vi "RTS Client.vi"() -> ()   [LabVIEW 2016]
uses:
  Type Definitions/RTS TDMS Filename Locations.ctl
  Type Definitions/RTS Save References.ctl
  Type Definitions/RTS Configuration Setup.ctl
  Type Definitions/RTS Wago Config.ctl
  Type Definitions/RTS APLUS Config.ctl
  Type Definitions/RTS Yokogawa MX Config.ctl
  Type Definitions/RTS Replay Server Control.ctl
  Type Definitions/RTS Server Configuration.ctl
  Type Definitions/RTS Station Settions TCP Comms.ctl
  Type Definitions/RTS Chamber Save Status.ctl
  Type Definitions/RTS Test Pattern.ctl
  Drivers/WAGO 750-881/Type Definitions/Wago Door Settings.ctl
  Drivers/WAGO 750-881/Type Definitions/Wago Door Relays By Station.ctl
  Drivers/WAGO 750-881/Type Definitions/Wago Door Operation.ctl
  Type Definitions/RTS Enable Door Openers.ctl
  Drivers/WAGO 750-881/Type Definitions/Wago Ground Leakage Relays.ctl
  Drivers/WAGO 750-881/Type Definitions/Wago Ground Leakage.ctl
  Drivers/WAGO 750-881/Type Definitions/Wago Polarity Selector Relays.ctl
  Drivers/WAGO 750-881/Type Definitions/Wago Polarity Selector.ctl
  Type Definitions/RTS Frequency Selector.ctl
  Drivers/WAGO 750-881/Type Definitions/Wago Room Enable.ctl
  Drivers/WAGO 750-881/Type Definitions/Wago Room Run.ctl
  Type Definitions/RTS Chamber Temperature Humidity Control.ctl
  Utility/Save File/File Setup (Public)/Type Definition/Save File DOE File Path Control.ctl
  Utility/Save File/File Setup (Public)/Type Definition/Save File DOE Data Save Filepaths.ctl
  Type Definitions/RTS Room Selector.ctl
  Type Definitions/RTS Reset Watt Hours.ctl
  Drivers/WAGO 750-881/Type Definitions/Wago Door Relays.ctl
  Drivers/WAGO 750-881/Type Definitions/Wago Contactor Settings.ctl
  Type Definitions/RTS TCP Commands.ctl
  Type Definitions/RTS TCP Multiple Connections Data.ctl
  Utility/Save File/File Setup (Public)/Type Definition/Save File DOE Configuration State.ctl
  Utility/Save File/File Setup (Public)/Type Definition/Save File DOE LabView Program.ctl
  Type Definitions/RTS Select System Number.ctl
  Utility/Save File/File Setup.lvlib
panel:
  in  "Custom CMD State":string
  in  "Test Setup":bool
  in  "Room Status":i32[](listbox)
  in  "Tree Selection":T1="Select Room/Stall"
  in  "Tab Control 3":enum32{"Page 1", "Page 2", "Page 3"}(tab)
  out "Start UI Loop":bool
  out "Raw Command":string
  in  "Filepath":T2
  out "Base Path":path
  out "Setup Info":string
  out "Data File Path":path
  out "Latest Save State":bool
  in  "Room OK?":T4
  in  "Room Run":T5
  out "Chamber Data":string[][](array[string])
  out "System Exit":bool=TRUE
  out "Control Exit":bool=TRUE
  out "Debug array 2":string[](array[string])
  in  "Debug?":bool
  out "Debug array":string[](array[string])
  out "Test Selected?":bool
  out "Point File Selected?":bool
  out "File Name Selected?":bool
  out "Deselect Log Data":bool=TRUE
  out "RTS Config Setup Output":T6
  in  "Tab Control 2":T15(tab)
  out "Chamber 1 Socket":string[][](array[string])
  out "Chamber 2 Socket":string[][](array[string])
  out "Chamber 3 Socket":string[][](array[string])
  out "Chamber 4 Socket":string[][](array[string])
  out "File  Version":string="Parametric Stand"
  in  "Save Data":bool
  out "Point File Path":path
  out "Error Out":errorcluster
  in  "Error In":errorcluster
  in  "Multicolumn Listbox":i32[](listbox)
  in  "Server Closed":string="The server VI closed the connection."
  in  "Configure Point File":bool
  in  "Setup Test":bool
  in  "Tab Control":T16(tab)
  out "Mixed Signal Graph 2":T17(graph)
  out "Tree Selection Display":string
  out "Save Status":T13
  in  "Wh Reset 8":T18 caption="Wh Reset"
  in  "Frequency 8":T19 caption="Frequency" items=["60 Hz", "50 Hz"]
  in  "Voltage 8":dbl caption="Voltage"
  in  "Wh Reset 7":T18 caption="Wh Reset"
  in  "Frequency 7":T19 caption="Frequency" items=["60 Hz", "50 Hz"]
  in  "Voltage 7":dbl caption="Voltage"
  in  "Wh Reset 6":T18 caption="Wh Reset"
  in  "Frequency 6":T19 caption="Frequency" items=["60 Hz", "50 Hz"]
  in  "Voltage 6":dbl caption="Voltage"
  in  "Wh Reset 5":T18 caption="Wh Reset"
  in  "Frequency 5":T19 caption="Frequency" items=["60 Hz", "50 Hz"]
  in  "Voltage 5":dbl caption="Voltage"
  in  "Wh Reset 4":T18 caption="Wh Reset"
  in  "Frequency 4":T19 caption="Frequency" items=["60 Hz", "50 Hz"]
  in  "Voltage 4":dbl caption="Voltage"
  in  "Wh Reset 3":T18 caption="Wh Reset"
  in  "Frequency 3":T19 caption="Frequency" items=["60 Hz", "50 Hz"]
  in  "Voltage 3":dbl caption="Voltage"
  in  "Wh Reset 2":T18 caption="Wh Reset"
  in  "Frequency 2":T19 caption="Frequency" items=["60 Hz", "50 Hz"]
  in  "Voltage 2":dbl caption="Voltage"
  in  "Wh Reset 1":T18 caption="Wh Reset"
  in  "Frequency":T19 items=["60 Hz", "50 Hz"]
  in  "Voltage":dbl
  in  "Station Voltage Send 5":bool
  in  "Station Voltage Send 1":bool
  in  "Station Voltage Send 6":bool
  in  "Station Voltage Send 2":bool
  in  "Station Voltage Send 7":bool
  in  "Station Voltage Send 3":bool
  in  "Station Voltage Send 8":bool
  in  "Station Voltage Send 4":bool
  in  "Polarity Selector":T20
  in  "Ground Leak Relays":T22
  out "Current Contactor Settings":T24
  out "Current Door Output Relays Status":T25
  in  "Station 8 CMD":bool
  in  "Station 7 CMD":bool
  in  "Station 6 CMD":bool
  in  "Station 5 CMD":bool
  in  "Station 4 CMD":bool
  in  "Station 3 CMD":bool
  in  "Station 2 CMD":bool
  in  "Station 1 CMD":bool
  in  "Door Settings":T26={"Station 1"={"Freezer"=enum."Clear Time Close Door", "Cab"=enum."Clear Time Close Door", "Slide"=enum."Clear Time Close Door"}, "Station 2"={"Freezer"=enum."Clear Time Close Door", "Cab"=enum."Clear Time Close Door", "Slide"=enum."Clear Time Close Door"}, "Station 3"={"Freezer"=enum."Clear Time Close Door", "Cab"=enum."Clear Time Close Door", "Slide"=enum."Clear Time Close Door"}, "Station 4"={"Freezer"=enum."Clear Time Close Door", "Cab"=enum."Clear Time Close Door", "Slide"=enum."Clear Time Close Door"}, "Station 5"={"Freezer"=enum."Clear Time Close Door", "Cab"=enum."Clear Time Close Door", "Slide"=enum."Clear Time Close Door"}, "Station 6"={"Freezer"=enum."Clear Time Close Door", "Cab"=enum."Clear Time Close Door", "Slide"=enum."Clear Time Close Door"}, "Station 7"={"Freezer"=enum."Clear Time Close Door", "Cab"=enum."Clear Time Close Door", "Slide"=enum."Clear Time Close Door"}, "Station 8"={"Freezer"=enum."Clear Time Close Door", "Cab"=enum."Clear Time Close Door", "Slide"=enum."Clear Time Close Door"}, "Door Enable"=enum."Enable Door Openers"}
  in  "Room Setpoints":T30={"Room Setpoint Temperature (*RM Dry Set P1)"=90.0, "Room Setpoint Humidity (*RM Hum Set P1)"=20.0, "Room Cool Temperature (*RM Cool Setp 1)"=65.0, "Room Dehum Temperature (*RM De Hum Set P1)"=60.0} {"Room Dehum Temperature (*RM De Hum Set P1)" min=30.0 max=120.0; "Room Cool Temperature (*RM Cool Setp 1)" min=30.0 max=120.0; "Room Setpoint Humidity (*RM Hum Set P1)" min=5.0 max=98.0; "Room Setpoint Temperature (*RM Dry Set P1)" min=40.0 max=120.0}
  in  "Update Room Setpoint":bool
  in  "CSV Data Save":T31={"CSV File Location"=path "C:/Technology Lab/NI-2010/Trunk/Refrigeration/RTS/System_Test_Data1.tdms", "CSV File Location 2"=path "C:/Technology Lab/NI-2010/Trunk/Refrigeration/RTS/System_Test_Data1.tdms", "CSV File Location 3"=path "", "CSV File Location 4"=path "", "CSV File Location 5"=path "", "CSV File Location 6"=path "", "CSV File Location 7"=path "", "CSV File Location 8"=path "", "Save References"={"CSV 1"=refnum, "CSV 2"=refnum, "CSV 3"=refnum, "CSV 4"=refnum, "CSV 5"=refnum, "CSV 6"=refnum, "CSV 7"=refnum, "CSV 8"=refnum}}
  in  "Update Plot":bool
  # "Refrigeration Test System"
  # "Voltage, Frequency & Watt Hour Selection"
  # "Station 1"
  # "Station 5"
  # "Station 2"
  # "Station 6"
  # "Station 3"
  # "Station 7"
  # "Station 4"
  # "Station 8"
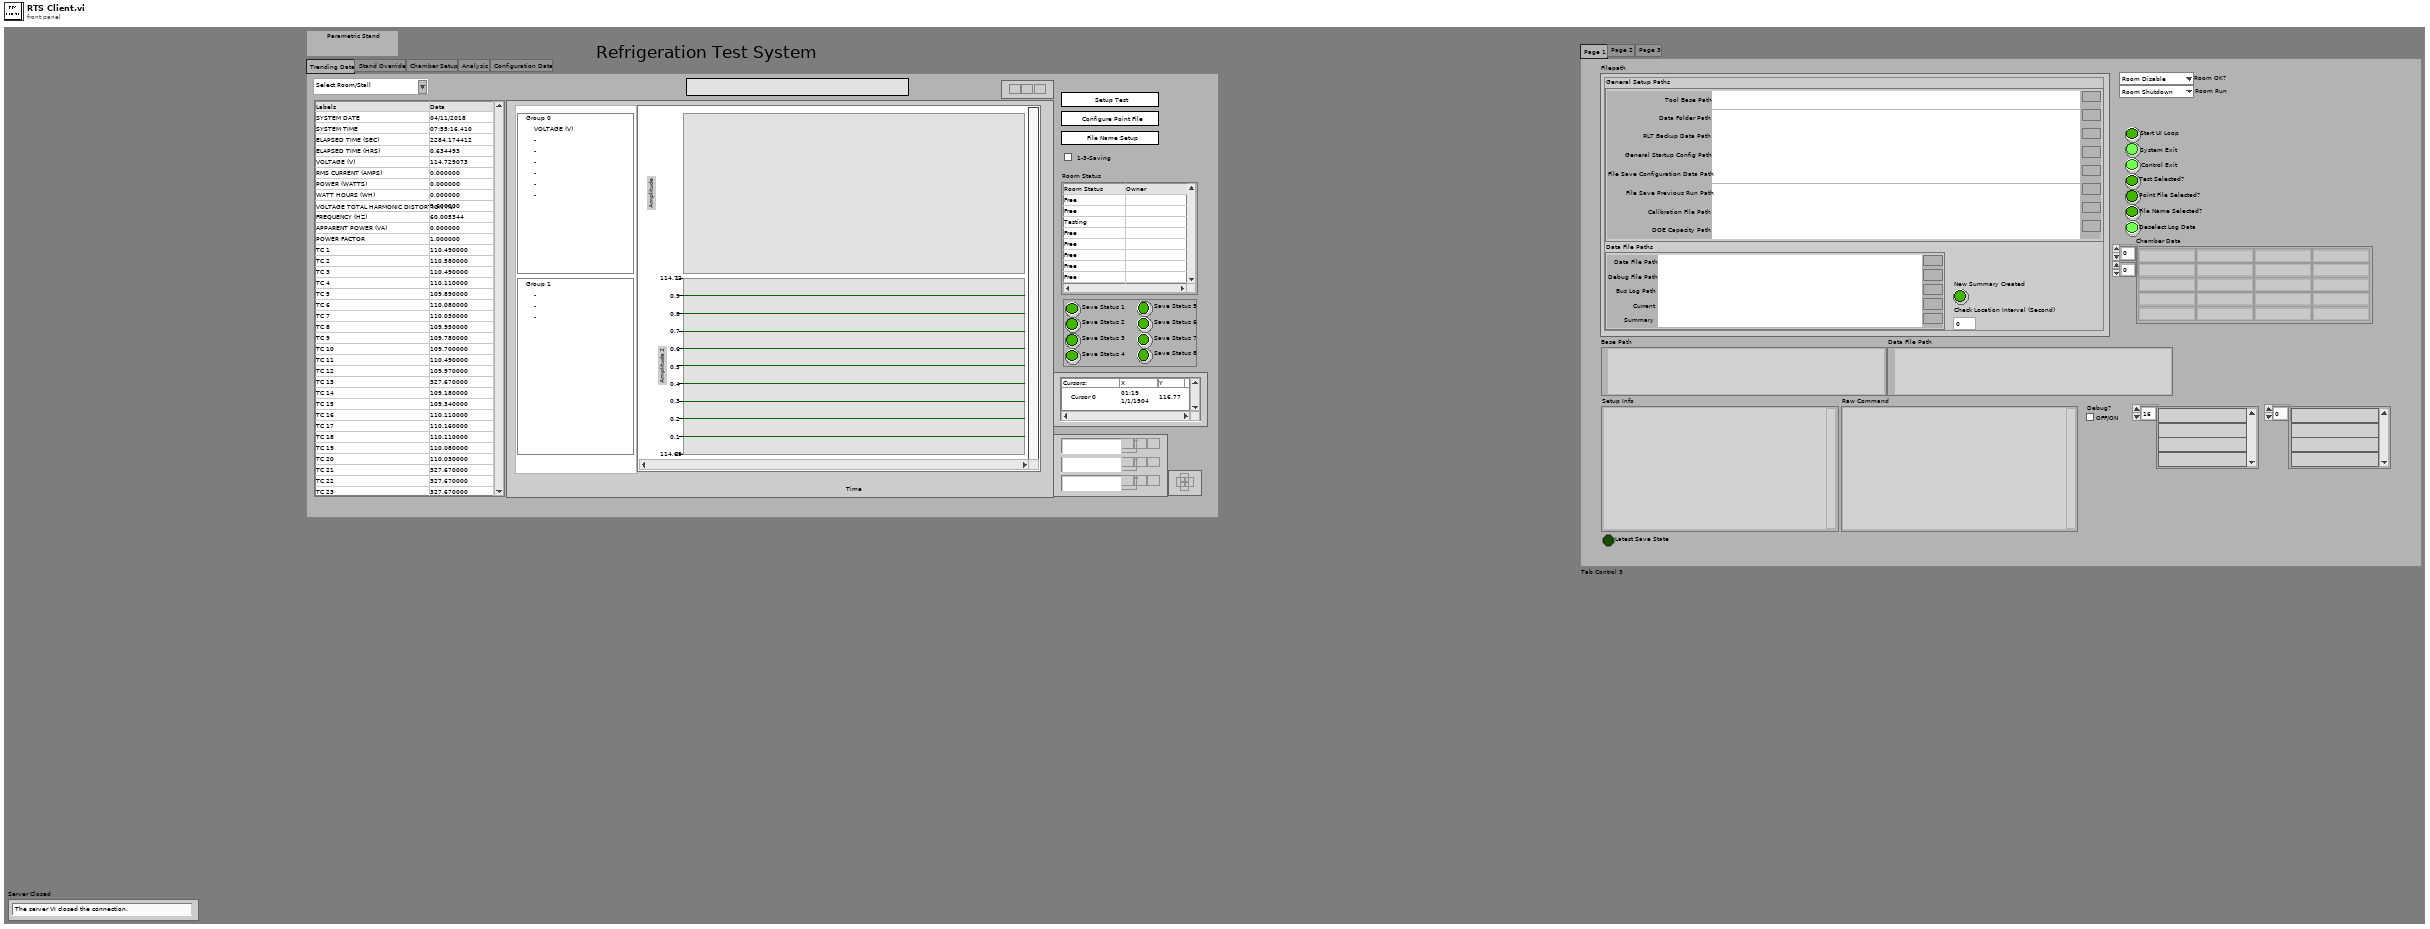
[diagram p1: front panel]
types:
  T1 = typedef "RTS Room Selector.ctl" = string
  T2 = typedef "File Setup.lvlib/Save File DOE File Path Control.ctl" = cluster{"General Setup Paths":cluster{"Calibration File Path":path, "DOE Capacity Path":path, "Data Folder Path":path, "RLT Backup Data Path":path, "Tool Base Path":path, "General Startup Config Path":path, "File Save Previous Run Path":path, "File Save Configuration Data Path":path}, "Data File Paths":T3, "New Summary Created":bool, "Check Location Interval (Second)":i32}
  T3 = typedef "File Setup.lvlib/Save File DOE Data Save Filepaths.ctl" = cluster{"Data File Path":path, "Debug File Path":path, "Bus Log Path":path, "Current":path, "Summary":path}
  T4 = typedef "Wago Room Enable.ctl" = enum16{"Room Disable", "Room OK"}
  T5 = typedef "Wago Room Run.ctl" = enum16{"Room Shutdown", "Room Run"}
  T6 = typedef "RTS Configuration Setup.ctl" = cluster{"Wago RTS":T7, "APLUS Array":T8[], "Yokogawa MX100 RTS Array":T9[], "Replay Server":T10[], "Server Configuration Array":T11[], "Station Settings":T12}
  T7 = typedef "RTS Wago Config.ctl" = cluster{"Disable":u16, "Interval":u16, "Controller":u16, "Address":u16, "IP Address":string, "AtoDmax":u16, "FullScale":u16, "VoltageType":u16, "Window1":u16, "Control1":u16, "Window2":u16, "Control2":u16}
  T8 = typedef "RTS APLUS Config.ctl" = cluster{"Disable":u16, "IP Address":string, "Input (4 Wire Unbalanced Load)":u16, "Dual Input (L1 115V, L2 230V)":u16, "LowLeakLimit":dbl, "Voltage Type":u16}
  T9 = typedef "RTS Yokogawa MX Config.ctl" = cluster{"IP Address":string, "TC Type":string, "Interval":u16, "Single Range":u16, "CalcWh":u16}
  T10 = typedef "RTS Replay Server Control.ctl" = cluster{"Interval":i16, "Repeat":u16, "Station":u16, "Load Path":path, "AutoMap":u16, "WattFactor":dbl, "AmpFactor":dbl}
  T11 = typedef "RTS Server Configuration.ctl" = cluster{"System":u16, "SysID":u16, "Title":string, "Enabled Server":u16, "Directory":string, "Configuration":string, "ValUpdate":u16, "TrendUpdate":u16, "ControlUpdate":u16, "Monitor":u16, "Pfact":u16, "Pipe":string, "TcpIP":u16, "Tunit":string, "ResultPath":path, "Door Sch DataLink":path, "MaxTCRate":u16, "Recovery":u16, "AutoRecovery":u16, "UsePowerFactor":u16, "OperatorPath":string, "Room":u16, "Station":u16, "Title":string, "DefMake":string, "Enabled Stall":u16, "Room":u16, "Title":string, "Station 1":u16, "Enabled 1":u16, "Station 2":u16, "Enabled 2":u16, "Station 3":u16, "Enabled 3":u16, "Station 4":u16, "Enabled 4":u16, "Station 5":u16, "Enabled 5":u16, "Station 6":u16, "Enabled 6":u16, "Station 7":u16, "Enabled 7":u16, "Station 8":u16, "Enabled 8":u16, "Title S1":string, "Title S2":string, "Title S3":string, "Title S5":string, "Title S6":string, "Title S7":string, "Title S8":string, "Title S4":string}
  T12 = typedef "RTS Station Settions TCP Comms.ctl" = cluster{"Point Files":cluster{"Point File 1":path, "Point File 2":path, "Point File 3":path, "Point File 4":path, "Point File 5":path, "Point File 6":path, "Point File 7":path, "Point File 8":path}, "Save Status":T13, "Setup Info":cluster{"Setup Info Station 1":string[][], "Setup Info Station 2":string[][], "Setup Info Station 3":string[][], "Setup Info Station 4":string[][], "Setup Info Station 5":string[][], "Setup Info Station 6":string[][], "Setup Info Station 7":string[][], "Setup Info Station 8":string[][]}, "Chamber Test Pattern":T14}
  T13 = typedef "RTS Chamber Save Status.ctl" = cluster{"Save Status 1":bool, "Save Status 2":bool, "Save Status 3":bool, "Save Status 4":bool, "Save Status 5":bool, "Save Status 6":bool, "Save Status 7":bool, "Save Status 8":bool}
  T14 = typedef "RTS Test Pattern.ctl" = cluster{" Pattern 1":path, "Pattern 2":path, "Pattern 3":path, "Pattern 4":path, "Pattern 5":path, "Pattern 6":path, "Pattern 7":path, "Pattern 8":path}
  T15 = enum32{"Chamber 1 Socket", "Chamber 2 Socket", "Chamber 3 Socket", "Chamber 4 Socket"}
  T16 = enum32{"Trending Data", "Stand Override", "Chamber Setup", "Analysis", "Configuration Data"}
  T17 = cluster{"Waveform Graph":waveform(dbl), "Waveform Graph":waveform(dbl), "Waveform Graph":waveform(dbl), "Waveform Graph":waveform(dbl), "Waveform Graph":waveform(dbl), "Waveform Graph":waveform(dbl), "Waveform Graph":waveform(dbl), "Waveform Graph":waveform(dbl), "Waveform Graph":waveform(dbl), "Waveform Graph":waveform(dbl)}
  T18 = typedef "RTS Reset Watt Hours.ctl" = enum16{"", "Reset Watt Hours"}
  T19 = typedef "RTS Frequency Selector.ctl" = u16
  T20 = typedef "Wago Polarity Selector Relays.ctl" = cluster{"Station 1":T21, "Station 2":T21, "Station 3":T21, "Station 4":T21, "Station 5":T21, "Station 6":T21, "Station 7":T21, "Station 8":T21}
  T21 = typedef "Wago Polarity Selector.ctl" = enum16{"Ground Neutral", "Ground Line"}
  T22 = typedef "Wago Ground Leakage Relays.ctl" = cluster{"Ground Leakage 1":T23, "Ground Leakage 2":T23, "Ground Leakage 3":T23, "Ground Leakage 4":T23, "Ground Leakage 5":T23, "Ground Leakage 6":T23, "Ground Leakage 7":T23, "Ground Leakage 8":T23}
  T23 = typedef "Wago Ground Leakage.ctl" = enum16{"0 - Normal GL", "1 - Measure GL"}
  T24 = typedef "Wago Contactor Settings.ctl" = cluster{"Station 1":cluster{"60 Hz Power":bool, "50 Hz Power":bool, "120V Range":bool, "240V Range":bool, "Ground Line":bool, "Ground Neutral":bool, "Room OK":bool, "Ground Leakage":T23}, "Station 2":cluster{"60 Hz Power":bool, "50 Hz Power":bool, "120V Range":bool, "240V Range":bool, "Ground Line":bool, "Ground Neutral":bool, "Fault":bool, "Ground Leakage":T23}, "Station 3":cluster{"60 Hz Power":bool, "50 Hz Power":bool, "120V Range":bool, "240V Range":bool, "Ground Line":bool, "Ground Neutral":bool, "Room Heat":bool, "Ground Leakage":T23}, "Station 4":cluster{"60 Hz Power":bool, "50 Hz Power":bool, "120V Range":bool, "240V Range":bool, "Ground Line":bool, "Ground Neutral":bool, "Room Blower":bool, "Ground Leakage":T23}, "Station 5":cluster{"60 Hz Power":bool, "50 Hz Power":bool, "120V Range":bool, "240V Range":bool, "Ground Line":bool, "Ground Neutral":bool, "Spare":bool, "Ground Leakage":T23}, "Station 6":cluster{"60 Hz Power":bool, "50 Hz Power":bool, "120V Range":bool, "240V Range":bool, "Ground Line":bool, "Ground Neutral":bool, "Room Pump":bool, "Ground Leakage":T23}, "Station 7":cluster{"60 Hz Power":bool, "50 Hz Power":bool, "120V Range":bool, "240V Range":bool, "Ground Line":bool, "Ground Neutral":bool, "Spare":bool, "Ground Leakage":T23}, "Station 8":cluster{"60 Hz Power":bool, "50 Hz Power":bool, "120V Range":bool, "240V Range":bool, "Ground Line":bool, "Ground Neutral":bool, "Spare":bool, "Ground Leakage":T23}}
  T25 = typedef "Wago Door Relays.ctl" = cluster{"Station 1 Freezer":bool, "Station 1 Cab":bool, "Station 1 Slide":bool, "Station 2 Freezer":bool, "Station 2 Cab":bool, "Station 2 Slide":bool, "Station 3 Freezer":bool, "Station 3 Cab":bool, "Station 3 Slide":bool, "Station 4 Freezer":bool, "Station 4 Cab":bool, "Station 4 Slide":bool, "Station 5 Freezer":bool, "Station 5 Cab":bool, "Station 5 Slide":bool, "Station 6 Freezer":bool, "Station 6 Cab":bool, "Station 6 Slide":bool, "Station 7 Freezer":bool, "Station 7 Cab":bool, "Station 7 Slide":bool, "Station 8 Freezer":bool, "Station 8 Cab":bool, "Station 8 Slide":bool, "Door Opener Enable":bool}
  T26 = typedef "Wago Door Settings.ctl" = cluster{"Station 1":T27, "Station 2":T27, "Station 3":T27, "Station 4":T27, "Station 5":T27, "Station 6":T27, "Station 7":T27, "Station 8":T27, "Door Enable":T29}
  T27 = typedef "Wago Door Relays By Station.ctl" = cluster{"Freezer":T28, "Cab":T28, "Slide":T28}
  T28 = typedef "Wago Door Operation.ctl" = enum16{"Clear Time Close Door", "Open Door", "Close Door", "PLC Timed Door Op"}
  T29 = typedef "RTS Enable Door Openers.ctl" = enum16{"Disable Door Openers", "Enable Door Openers"}
  T30 = typedef "RTS Chamber Temperature Humidity Control.ctl" = cluster{"Room Setpoint Temperature (*RM Dry Set P1)":dbl, "Room Setpoint Humidity (*RM Hum Set P1)":dbl, "Room Cool Temperature (*RM Cool Setp 1)":dbl, "Room Dehum Temperature (*RM De Hum Set P1)":dbl}
  T31 = typedef "RTS TDMS Filename Locations.ctl" = cluster{"CSV File Location":path, "CSV File Location 2":path, "CSV File Location 3":path, "CSV File Location 4":path, "CSV File Location 5":path, "CSV File Location 6":path, "CSV File Location 7":path, "CSV File Location 8":path, "Save References":T32}
  T32 = typedef "RTS Save References.ctl" = cluster{"CSV 1":refnum<file>, "CSV 2":refnum<file>, "CSV 3":refnum<file>, "CSV 4":refnum<file>, "CSV 5":refnum<file>, "CSV 6":refnum<file>, "CSV 7":refnum<file>, "CSV 8":refnum<file>}
  T33 = typedef "RTS TCP Commands.ctl" = string
  T34 = enum8{"Enabled", "Disabled", "Disabled and Grayed Out"}
  T35 = typedef "File Setup.lvlib/Save File DOE LabView Program.ctl" = enum16{"No Name Found", "DOE Stand", "Dishwasher Kitchen", "Portable Stand", "HEWH", "Dryer", "Dryer WILT", "HCC", "PRAT", "HEWH RLT", "Refrigeration", "Gas Water Heater"}
  T36 = typedef "File Setup.lvlib/Save File DOE Configuration State.ctl" = enum16{"Open Front Panel", "Load Config"}
  T37 = enum32{"invalid app kind", "Development System", "Run Time System", "Student Edition", "Embedded LabVIEW", "Evaluation", "Custom"}
  T38 = enum32{"Invalid", "Standard", "Closed", "Hidden", "Minimized", "Maximized"}
  T39 = typedef "DOE Main Control.ctl" = cluster{"Test Fixture Hardware":T40, "GEA2":T50, "DOE Capacity Measurments":T51, "Initialize.Washer In":T52}
  T40 = typedef "DOE Test Fixture Hardware.ctl" = cluster{"Power ":T41, "Weight Scale":cluster{"Com Options":T42, "Select Scale":string}, "Flow Rates":cluster{"Laurel Cold IP Address":string, "Laurel Hot IP Address":string, "Hot Water Laurel VISA":refnum<visa-resource-name>, "Cold Water Laurel VISA":refnum<visa-resource-name>, "Remote Port":u16, "Laurel Communication Type":string, "Meters To Collect (Hot Cold)":string, "HOT Laurel Reference":refnum<k5>, "COLD Laurel Reference":refnum<k5>}, "Analog Data":cluster{"Agilent":cluster{"Agilent 34972_1":refnum<visa-resource-name>, "Agilent 34972_2":refnum<visa-resource-name>, "Agilent 34972_3":refnum<visa-resource-name>, "Agilent 34972_4":refnum<visa-resource-name>, "Agilent 34972_5":refnum<visa-resource-name>, "Agilent 34972_6":refnum<visa-resource-name>, "Agilent Gain":dbl, "TC Type (K,J,T)":string, "Instrument IDN?":string, "TC Channels-List":string, "Analog Channels-List":string, "Agilent Cluster Array":T43[], "TC Channels-List 2":string, "Analog Channels-List 2":string}, "Yokogawa":cluster{"MW100":refnum<visa-resource-name>, "Intellifaucet":bool}, "Select Analog":string, "TC Coefficients":T44, "NI Tasks (Dryer DOE)":refnum<k21>[], "Laurel Analog":cluster{"Laurel IP (Water Temp)":string, "Laurel IP (Pressure)":string}}, "ITHX-Temp Humidity":cluster{"IP Address 1":string, "Remote Port":u16, "IP Address 2":string, "IP Address 3":string}, "Gas Meter":T45, "Barometric Pressure":cluster{"HEISE 901A":refnum<visa-resource-name>, "Use Barometer?":bool}}
  T41 = typedef "UTILITY Power Inputs Control.ctl" = cluster{"Yokogawa":cluster{"WT210":cluster{"Sample Rate (1: 0.25s)":i32, "A Range (12: 20A)":i32, "V Range (6: 600V)":i32, "Power VISA Yokogawa WT210":refnum<visa-resource-name>}, "WT500":cluster{"Power VISA Yokogawa WT500":refnum<visa-resource-name>, "V Range (8: 1000V)":i32, "I Range (7: 40A)":i32, "Update Rate (3: 500ms)":i32}, "WT310_2":cluster{"Sample Rate (1: 0.25s)":i32, "A Range (12: 20A)":i32, "V Range (6: 600V)":i32, "Power VISA Yokogawa WT310_2":refnum<visa-resource-name>}, "WT310_3":cluster{"Sample Rate (1: 0.25s)":i32, "A Range (12: 20A)":i32, "V Range (6: 600V)":i32, "Power VISA Yokogawa WT310_3":refnum<visa-resource-name>}}, "Aplus":cluster{"Aplus IP Address":string, "Remote Port":i32, "Instrument":string, "Instr Driver Revision":string}, "Power Limits":cluster{"Crest Factor":cluster{"Upper Limit":dbl, "Lower Limit":dbl}, "Harmonic Content":cluster{"Uthd":dbl}, "Voltage":cluster{"% Error":dbl}, "Stability":cluster{"<1 Watt ":cluster{"Wattage":dbl, "Slope (mW/H)":dbl}, ">1 Watt":cluster{"1%Power/Hour":dbl}}}, "Nominal Voltage":i32, "Time Limit (s)":dbl, "Power Variation Limit (%)":dbl, "Power Supply":cluster{"Chroma 61605":refnum<visa-resource-name>, "Use Chroma?":bool}}
  T42 = typedef "IND560 Configuration.ctl" = cluster{"IND560Scale VISA":refnum<visa-resource-name>, "IP Address":string, "Remote Port":u16, "Setra Scale VISA":refnum<visa-resource-name>, "GSE 350":refnum<visa-resource-name>}
  T43 = typedef "HEWH Agilent Cluster.ctl" = cluster{"Label":string, "Agilent Channel":string, "Panel ID":string, "Source":string, "Temperature":dbl}
  T44 = typedef "UTILITY TC Coefficients.ctl" = cluster{"TC Coefficients 1":dbl[], "TC Coefficients 2":dbl[], "TC Coefficients 3":dbl[], "TC Coefficients 4":dbl[], "TC Coefficients 5":dbl[], "TC Coefficients 6":dbl[], "TC Coefficients 7":dbl[]}
  T45 = typedef "FMA1600A COM Ports.ctl" = cluster{"Gas Meter 1":refnum<visa-resource-name>, "Gas Meter 2":refnum<visa-resource-name>, "Gas Meter 3":refnum<visa-resource-name>, "Gas Meter 4":refnum<visa-resource-name>, "Gas Meter 5":refnum<visa-resource-name>, "Gas Meter 6":refnum<visa-resource-name>, "Data Frame Format":T46, "Measurement Data":T47, "Measurement Units":T48}
  T46 = typedef "Data Frame.ctl" = cluster{"Absolute Pressure":bool, "Gauge/Diff. Pressure":bool, "Barometric Pressure":bool, "Temperature":bool, "Volumetric":bool, "Mass":bool, "Setpoint":bool, "Valve Drive":bool, "Totalizer":bool, "Totalizer Timer":bool, "Totalizer Average Flow":bool, "Totalizer Peak Flow":bool, "Gas Selected":bool, "Tot. Timer Format":u16}
  T47 = typedef "Data Cluster.ctl" = cluster{"Absolute Pressure":dbl, "Gauge/Diff. Pressure":dbl, "Barometric Pressure":dbl, "Temperature":dbl, "Volumetric Flow":dbl, "Mass Flow":dbl, "Setpoint":dbl, "Valve Drive":dbl, "Totalizer":dbl, "[hr]":dbl, "[min]":dbl, "[sec]":dbl, "Totalizer Average Flow":dbl, "Totalizer Peak Flow":dbl, "Gas selected":string}
  T48 = typedef "FMA1600A Units String.ctl" = cluster{"Software Rev":string, "Model Number":string, "Manufacturer Info":string, "Software Sub-Rev":string, "Board Rev":string, "Units of Measure Input":T49}
  T49 = typedef "Units of Measure.ctl" = cluster{"Abs. Pressure":string, "Gauge/Diff. Press.":string, "Barometric Press.":string, "Temperature":string, "Volume":string, "Mass":string, "Setpoint":string, "Valve Drive":string, "Totalizer":string, "Tot. Timer":string, "Tot. Avg. Flow":string, "Tot. Peak Flow":string}
  T50 = typedef "GEA2.ctl" = cluster{"Address":u8, "Source":u8, "Viper/Hawk":u8}
  T51 = typedef "DOE Capacity Measurments.ctl" = cluster{"Weight 1":dbl, "Model Number 1":string, "Temp 1":dbl, "Serial Number 1":string, "Lab Number 1":string, "Lab Number 2":string, "Serial Number 2":string, "Temp 2":dbl, "Model Number 2":string, "Weight 2":dbl, "Lab Number 3":string, "Serial Number 3":string, "Temp 3":dbl, "Model Number 3":string, "Weight 3":dbl, "Lab Number 4":string, "Serial Number 4":string, "Temp 4":dbl, "Model Number 4":string, "Weight 4":dbl, "Capacity Measurment Output String":string[][]}
  T52 = typedef "Save File.lvlib/Save File Washer.ctl" = cluster{"Appliance Details":T53, "Display Data (RLT)":T59}
  T53 = typedef "File Setup.lvlib/Save File DISH Dishwasher Details.ctl" = cluster{"FileVersionInfo":T54, "Dishwasher Info":cluster{"Open Cup Weight (gm):":dbl, "Auto Cup Weight (gm):":dbl, "Detergent-Dish:":string, "Inlet Temperature-Dish:":string, "Cycle Mode-Dish:":string, "Unit Control-Dish:":string, "Manufacturer-Dish:":string}, "Washer Info":cluster{"Hot Water Temperature (Fahrenheit):":string, "Cold Water Temperature (Fahrenheit):":string, "Capacity (cu.ft):":dbl, "Initial Cloth Weight:":dbl, "Cloth Lot:":i32, "Model Family:":string, "Program Name:":string, "Cycle Selection:":string, "Wash Temperature:":string, "Rinse Temperature:":string, "Load Size:":string}, "File Name Output Array":string[][], "Calibration Output Array":string[][], "Appliance Common":T55, "Water Heater":cluster{"Heating Mode:":string}, "Dryer":cluster{"Heat Setting:":T56, "Washer Water Temperature (60 ± 5°F):":u16, "Water Hardness (PPM):":u16, "Dryness Setting:":T56, "Dryer Type:":string, "Exhaust:":string, "Drying Cycle:":string, "Load Type:":string, "Nominal Load Weight":string, "Dryer Initial IMC Data":T57}}
  T54 = typedef "FileVersionInformation.ctl" = cluster{"FileVersion":string, "ProductName":string, "InternalName":string, "CompanyName":string, "LegalCopyright":string, "FileDescription":string}
  T55 = typedef "DOE Appliance Common.ctl" = cluster{"Engineer:":string, "Model Number:":string, "Serial Number:":string, "Comments:":string, "Station ID:":string, "Technician:":string, "TR Number:":string, "Lab ID:":string, "Voltage:":string, "Water Pressure (PSI):":string, "Test Date:":string, "Computer Name:":string, "IP Address:":string, "Ambient RH:":string, "Frequency:":string, "Build:":string, "Filename:":string, "Test Type:":string, "Load Run #:":i32, "Ambient Temperature (F):":string, "File Path:":path, "Cycles Per Year":u32}
  T56 = typedef "Custom Pallet String.ctl" = string
  T57 = typedef "DPT IMC Data.ctl" = cluster{"Measured IMC (lbs)":dbl, "Actual Initial RMC (%)":dbl, "RMC (Desired %)":dbl, "Bone Dry Wt(lbs)":dbl, "Tolerance(%)":dbl, "Actual Final RMC (%)":dbl, "CEF (lbf/kWh)":dbl, "Minimum Weight (lbf)":dbl, "Average Weight (lbf)":dbl, "Maximum Weight (lbf)":dbl, "Measured IMC In Range?":bool, "Moisture Reduction Factor":dbl, "Field Use Factor":dbl, "Empty Dryer Cold Weigth":dbl, "Energy Standard":T58, "Weight Cloth (lbs)":dbl, "Relative Moisture Content (%)":dbl, "Relative Moisture Content - Avg (%)":dbl}
  T58 = typedef "DOE Dryer Standard.ctl" = enum16{"D2-Automatic Dryer", "D2-Timer Dryer", "D1-Automatic Dryer", "D1-Timer Dryer", "Other"}
  T59 = typedef "Save File Appliance Display.ctl" = cluster{"Status Color":u32, "Serial Number Display":string, "Cycle Count Display":i32, "Station Label Display":string, "Current Run Start Time Display":dbl, "Board ID Display":string, "RPM Display":u32, "Current Display":dbl, "Current Path Display":path, "Saving Display":bool, "Unit Type Display":T60, "Total Time On Display":dbl, "UI Button":bool}
  T60 = typedef "Save File.lvlib/Save File Unit Type.ctl" = enum32{"", "Viper", "Hawk", "2015"}
  T61 = cluster{"Core":cluster{"Current VI Reference":refnum<vi>, "Close Panel on Exit?":bool}, "Filepath":T2, "Test Selected?":bool, "Point File Selected?":bool, "File Name Selected?":bool}
  T62 = cluster{"Current VI Reference":refnum<vi>, "Close Panel on Exit?":bool}
  T63 = typedef "RTS TCP Multiple Connections Data.ctl" = cluster{"Clients":refnum<k5>[], "Listener":refnum<k5>, "Data Array":string[]}
  T64 = typedef "RTS Select System Number.ctl" = string
  T65 = cluster{"Core":cluster{"Current VI Reference":refnum<vi>, "Close Panel on Exit?":bool}, "ListBox Selection":i32[], "All Data":dbl[][], "Full Item Names":string[], "CSV Data Save":T31, "Data":T63, "Tree Selection":T1, "RTS Config Setup":T6, "Server Write Data":string, "Station Owner Names":string[], "Chamber Data":string[][], "Listbox Item Names":string[], "Custom Titles":string[], "Filepath":T2}
  T66 = typedef "RTS Voltage Frequency Settings.ctl" = cluster{"Voltage 1":dbl, "Voltage 2":dbl, "Voltage 3":dbl, "Voltage 4":dbl, "Voltage 5":dbl, "Voltage 6":dbl, "Voltage 7":dbl, "Voltage 8":dbl, "Frequency 1":T19, "Frequency 2":T19, "Frequency 3":T19, "Frequency 4":T19, "Frequency 5":T19, "Frequency 6":T19, "Frequency 7":T19, "Frequency 8":T19, "Ground Leak Relays":T22, "Polarity Selector":T20, "Room Setpoints":T30}
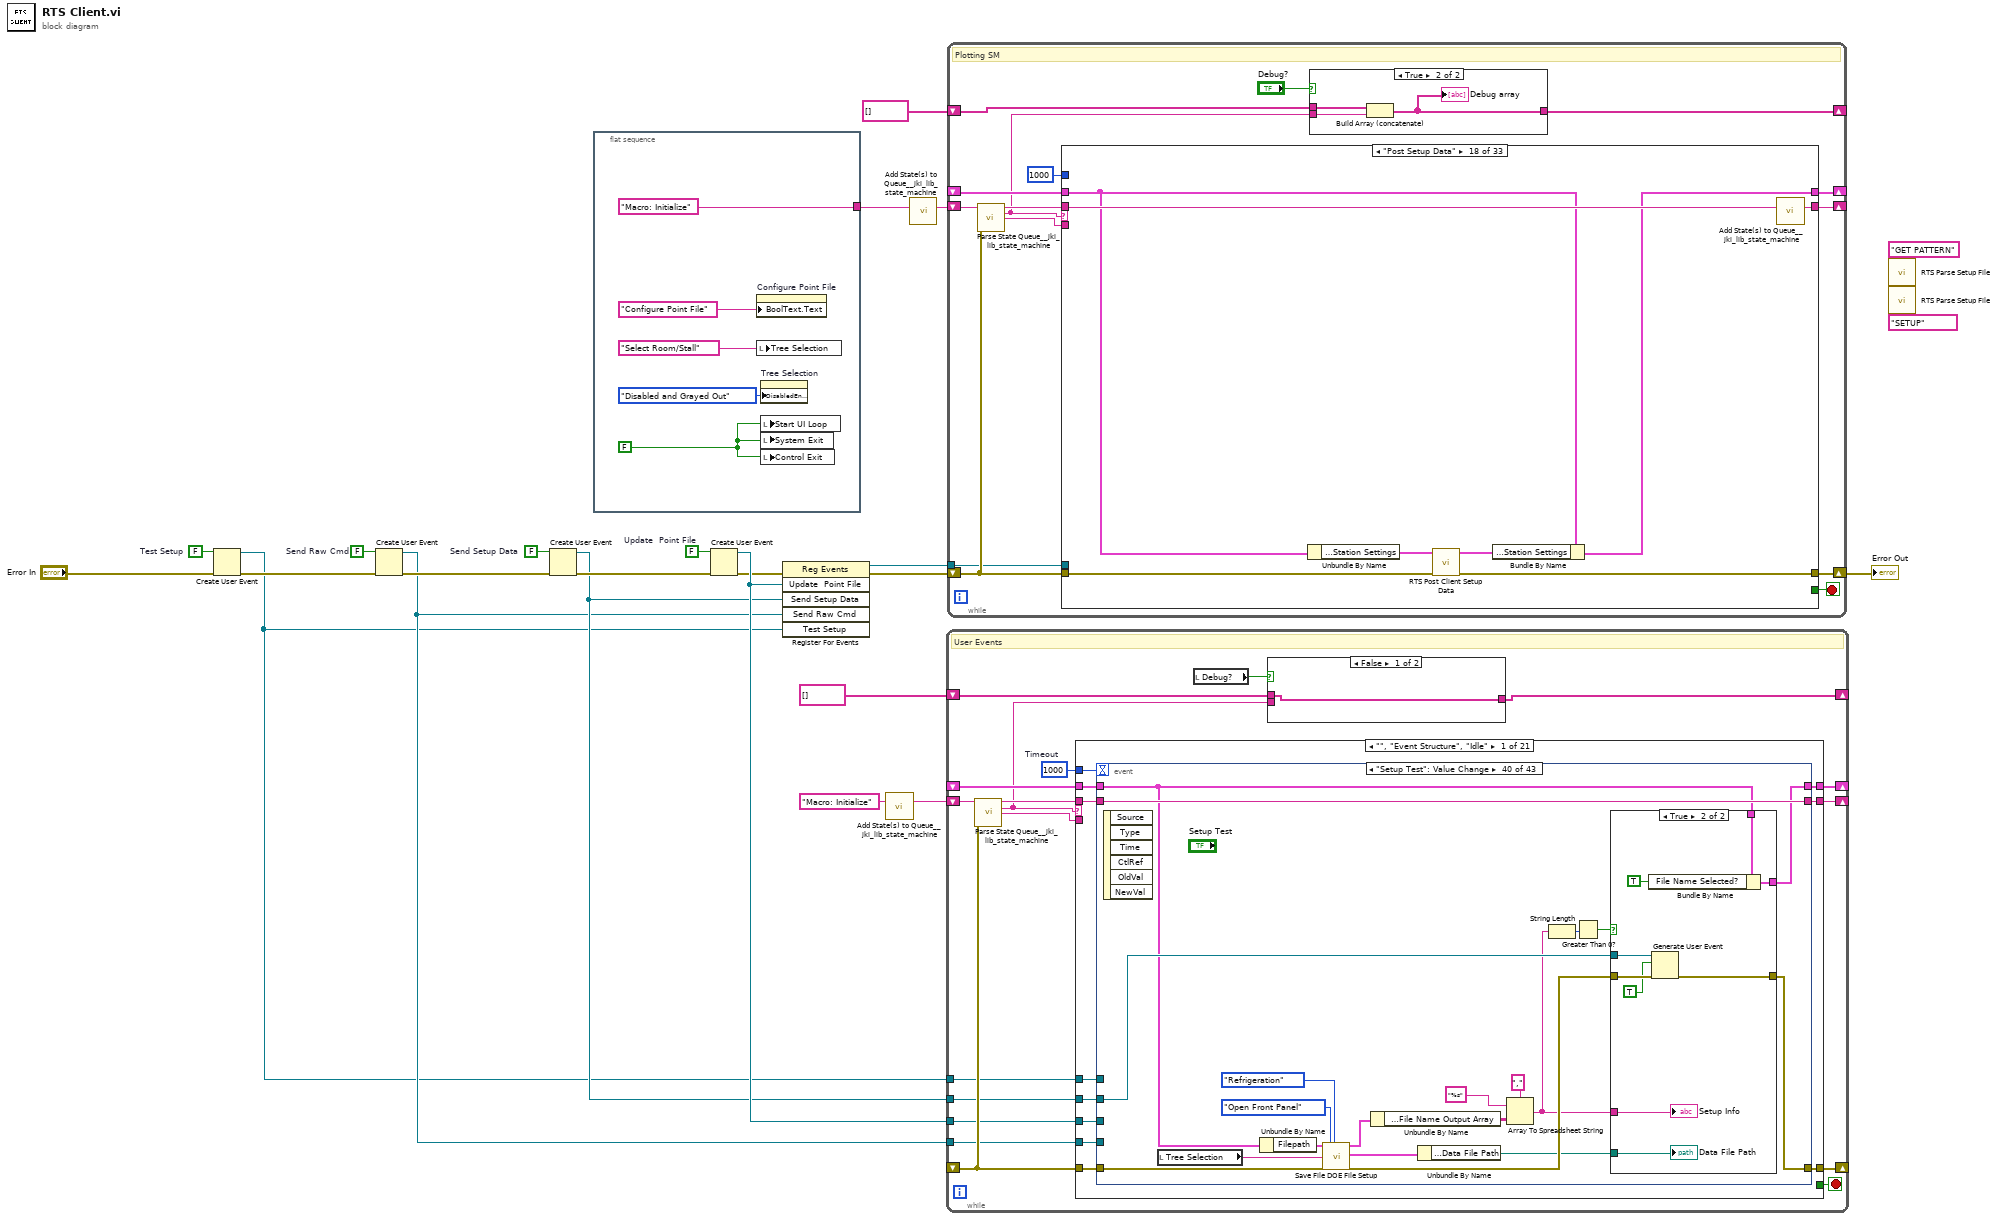
[diagram p0: block diagram]
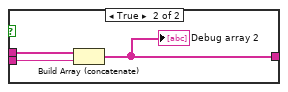
[diagram p2: hidden frame]
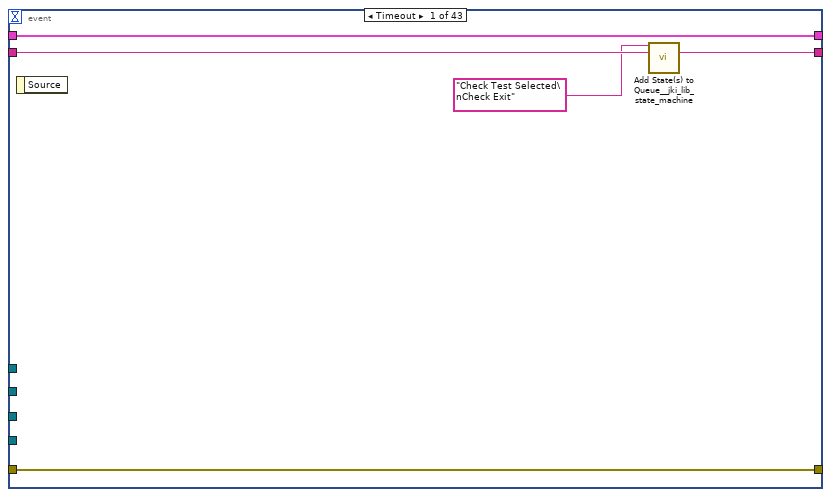
[diagram p3: hidden frame]
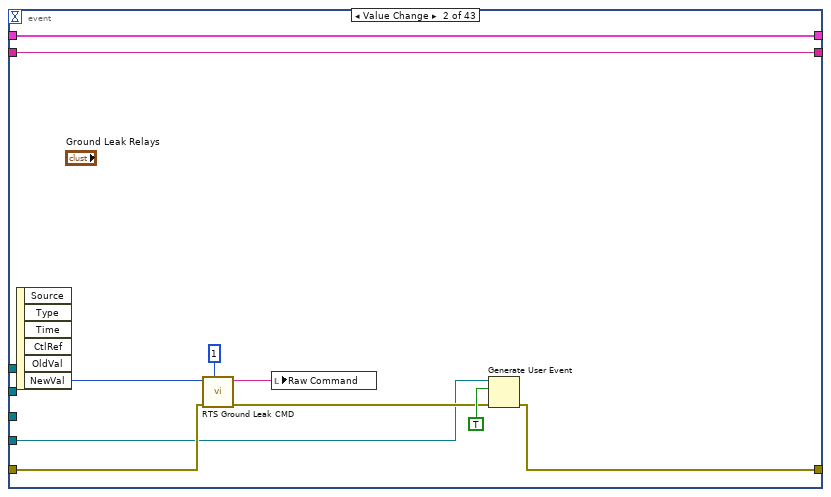
[diagram p4: hidden frame]
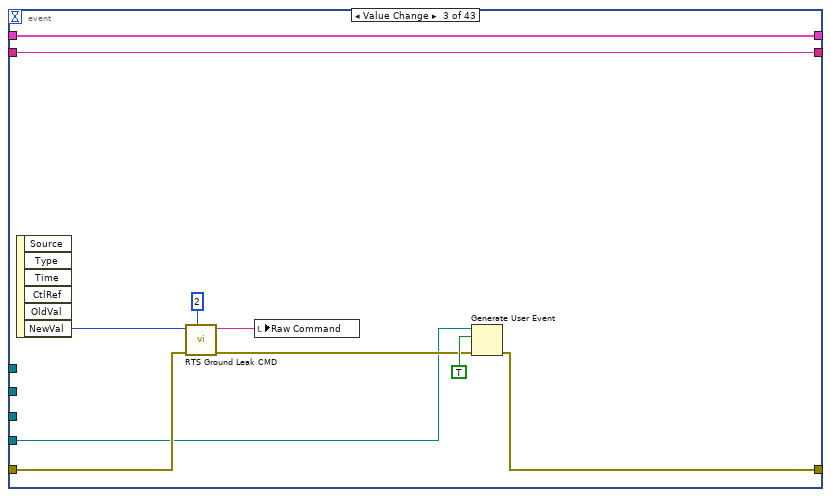
[diagram p5: hidden frame]
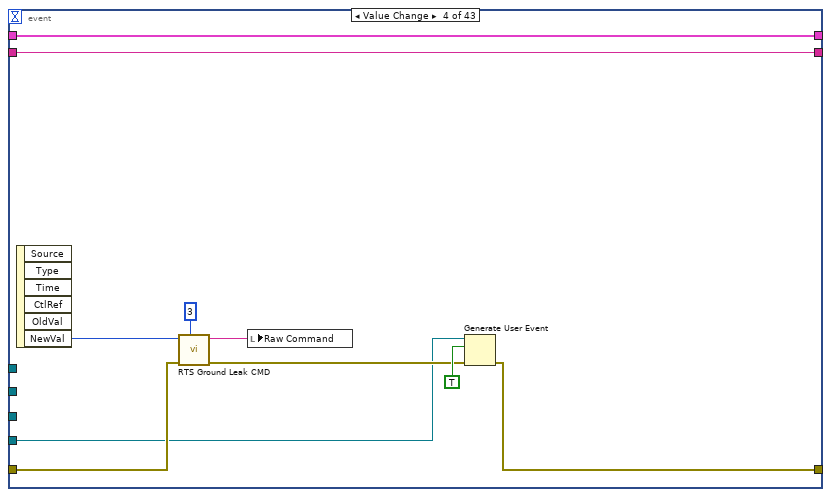
[diagram p6: hidden frame]
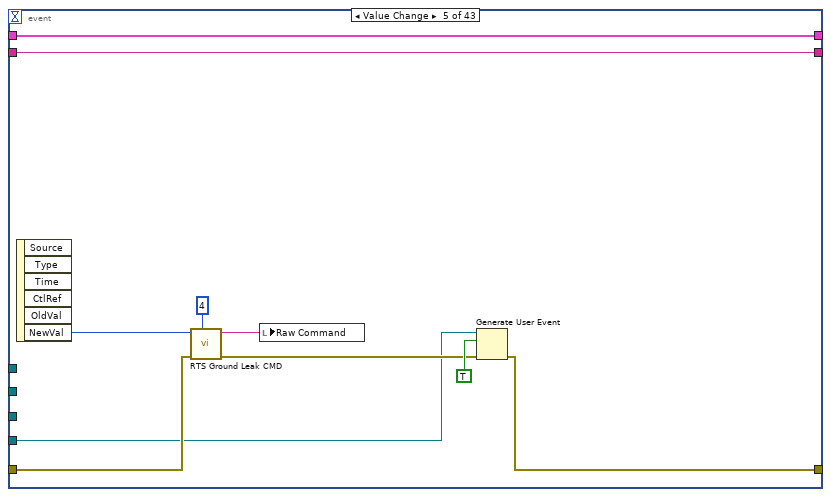
[diagram p7: hidden frame]
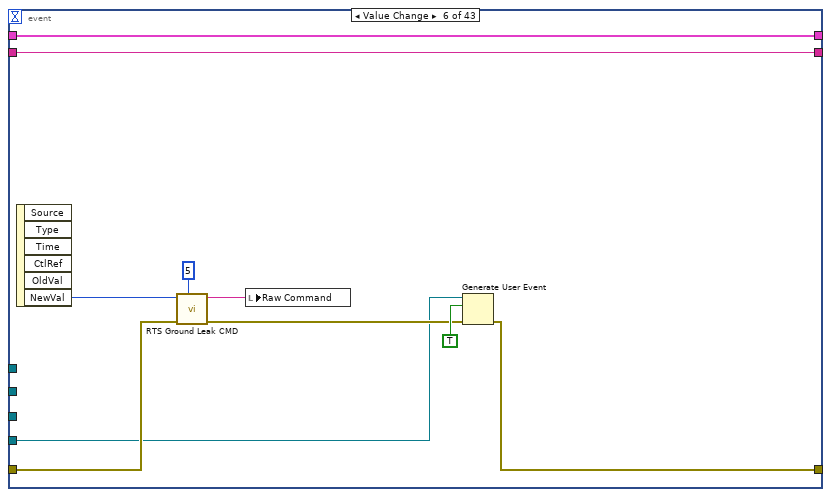
[diagram p8: hidden frame]
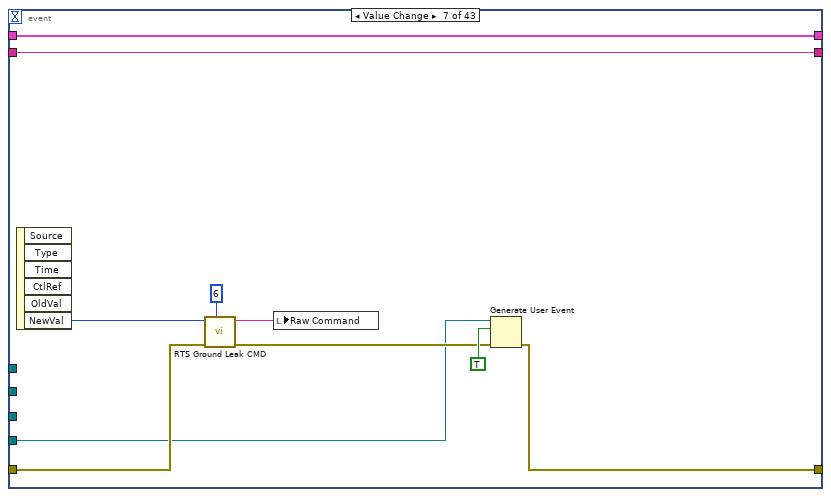
[diagram p9: hidden frame]
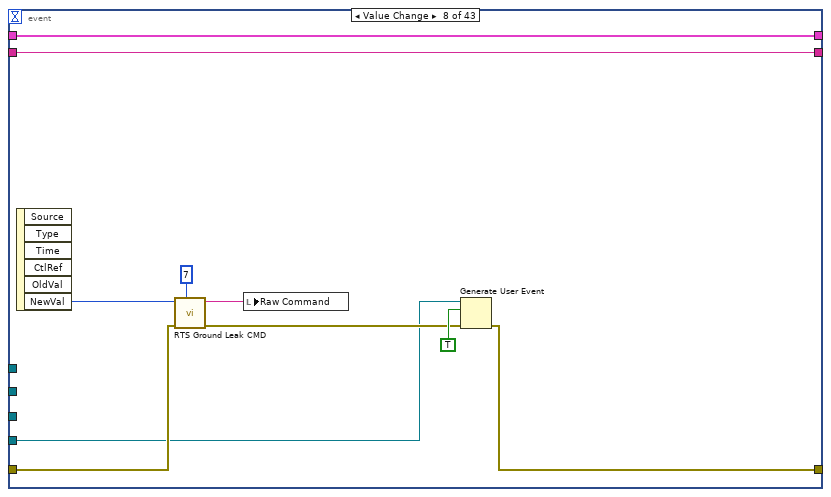
[diagram p10: hidden frame]
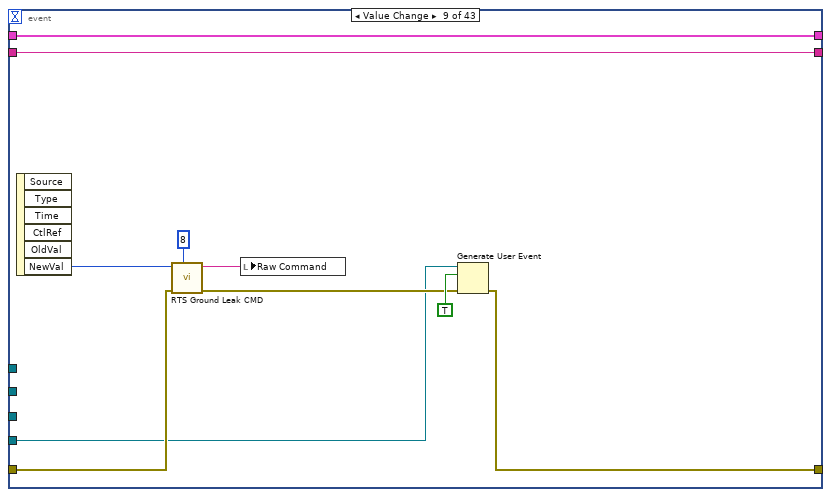
[diagram p11: hidden frame]
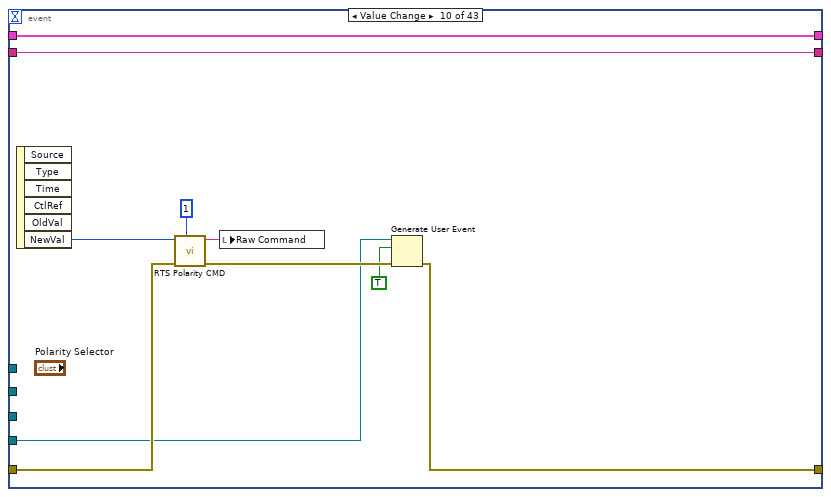
[diagram p12: hidden frame]
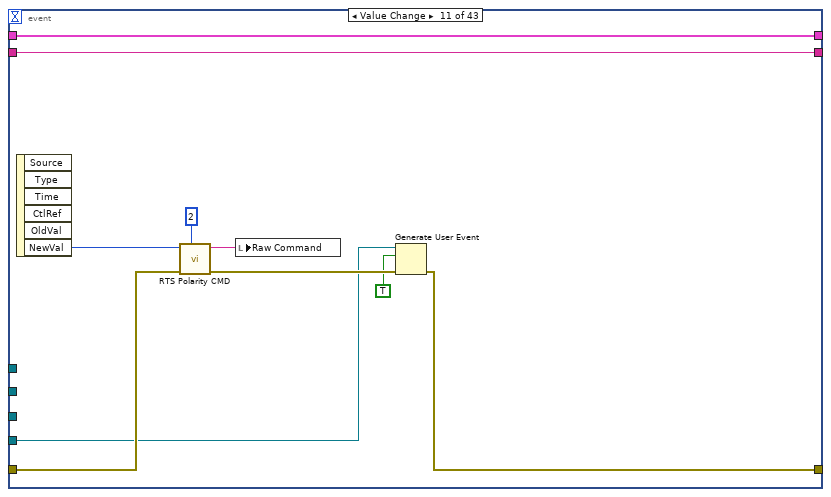
[diagram p13: hidden frame]
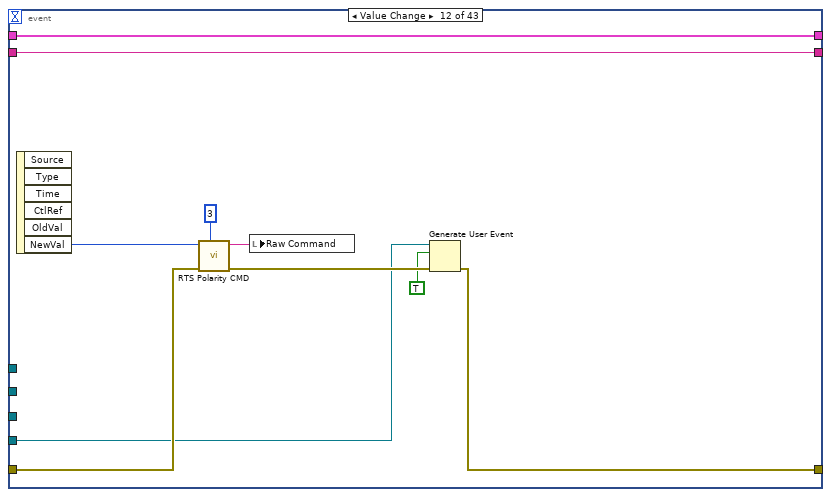
[diagram p14: hidden frame]
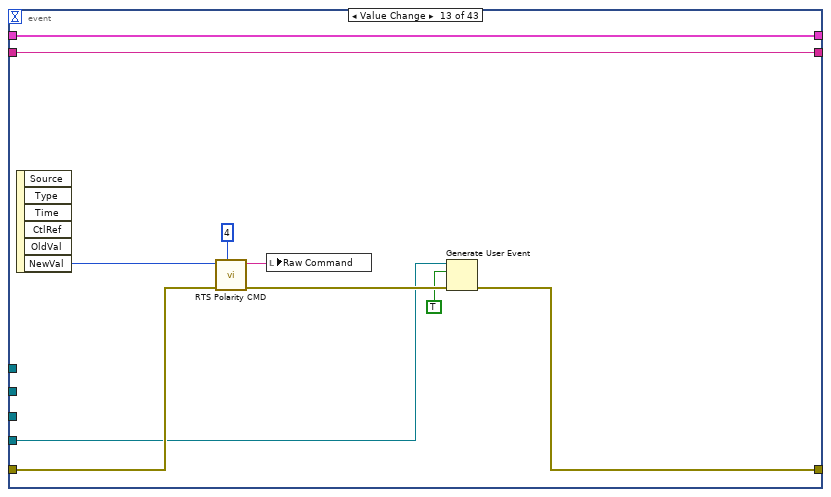
[diagram p15: hidden frame]
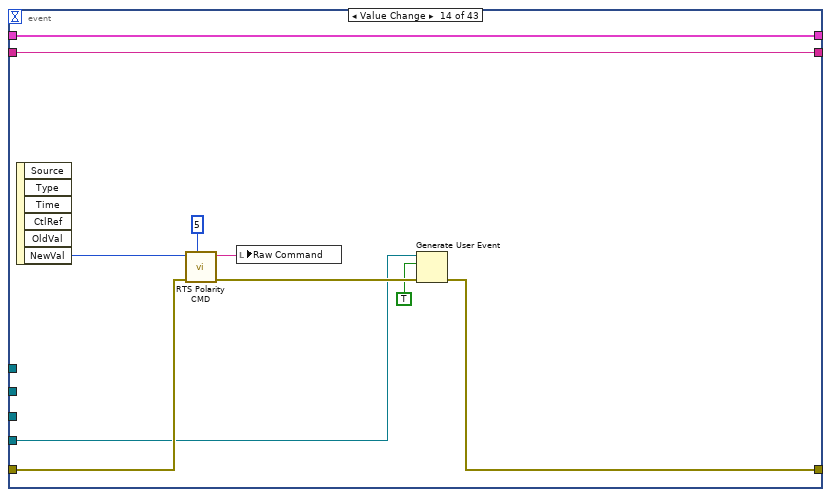
[diagram p16: hidden frame]
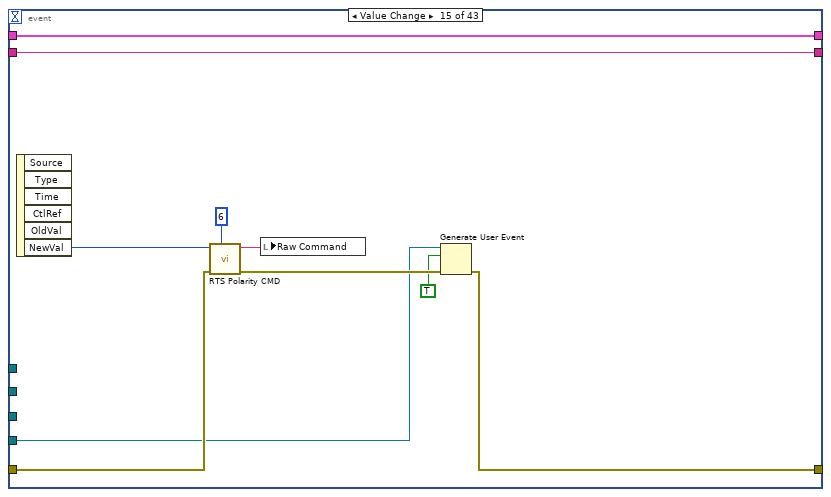
[diagram p17: hidden frame]
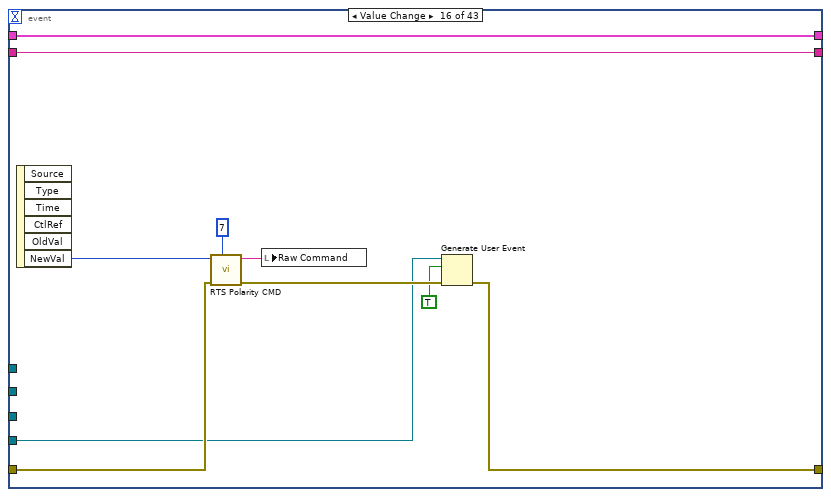
[diagram p18: hidden frame]
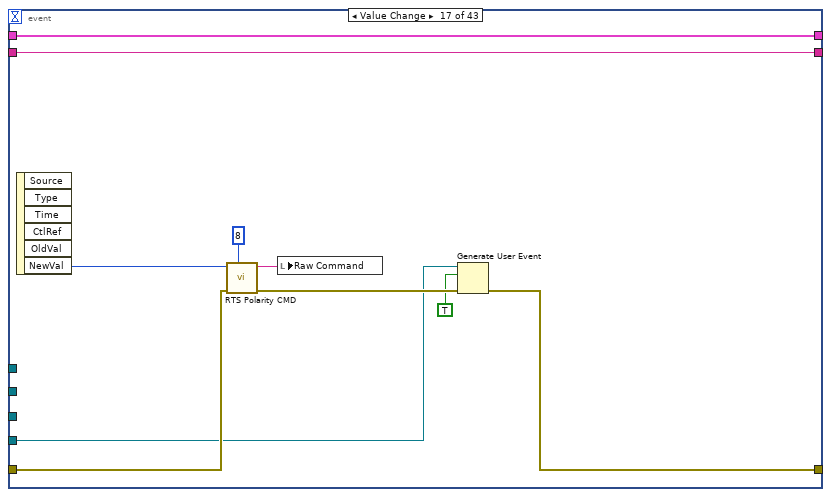
[diagram p19: hidden frame]
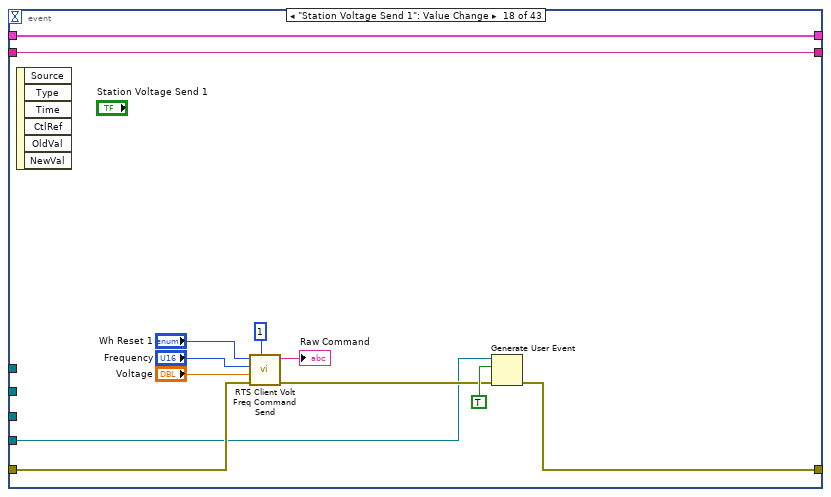
[diagram p20: hidden frame]
diagram:
  (unwired) T33 "SETUP" ("TCP Commands")
  (unwired) T33 "GET PATTERN" ("TCP Commands 2")
  w4 = FALSE  # Test Setup
  w7 = FALSE  # Send Raw Cmd
  w12 = FALSE  # Send Setup Data
  w16 = FALSE  # Update  Point File
  n1 = Create User Event(user event datatype=w4, error in="Error In") -> (user event=w1:refnum<user-event>, error out=w2:errorcluster)
  n2 = Create User Event(user event datatype=w7, error in=w2) -> (user event=w5:refnum<user-event>, error out=w6:errorcluster)
  n3 = Create User Event(user event datatype=w12, error in=w6) -> (user event=w9:refnum<user-event>, error out=w10:errorcluster)
  n4 = flat-sequence {
    tunnel: ["Macro: Initialize"] -> w21
    frame #0 {
      w23 = FALSE ("System Exit")
      n5 = property on="Configure Point File" class="Bool"("BoolText.Text"="Configure Point File" ("Boolean Text.Text")) -> ()  [unwired: 2 in, 2 out]
      n6 = local write "Tree Selection"(T1 "Select Room/Stall" ("Room Selection")) -> ()
      n7 = property on="Tree Selection" class="CmbBox (strict)"("DisabledEnum"=T34."Disabled and Grayed Out" ("Disabled")) -> ()  [unwired: 2 in, 2 out]
      n8 = local write "Start UI Loop"(w23) -> ()
      n9 = local write "System Exit"(w23) -> ()
      n10 = local write "Control Exit"(w23) -> ()
    }
  }
  n11 = Create User Event(user event datatype=w16, error in=w10) -> (user event=w13:refnum<user-event>, error out=w11:errorcluster)
  n12 = register-events(error in=w11, w13, w9, w5, w1) -> (reference out=w15:refnum<event-registration>, error out=w14:errorcluster)  [unwired: 1 in]
  n13 = call <vilib>:"Add State(s) to Queue__jki_lib_state_machine.vi"("State(s) in (\"\")"="Macro: Initialize") -> ("States Out"=w18:string)  [unwired: 14 in]
  n14 = call <vilib>:"Add State(s) to Queue__jki_lib_state_machine.vi"("State(s) in (\"\")"=w21) -> ("States Out"=w20:string)  [unwired: 14 in]
  n15 = while "UI Events" {
    shift-right: [w39] -> _
    shift-left: _ -> [w38]
    shift-right: [w42] -> _
    shift-left: _ -> [w36]
    shift-right: [w41] -> _
    shift-left: w18 -> [w43]
    tunnel: w13 -> [w35]
    tunnel: w9 -> [w34]
    shift-right: [w31] -> _
    shift-left: string[] [] -> [w33]
    tunnel: w5 -> [w29]
    tunnel: w1 -> [w28]
    stop <- w40 stop-if-true
    w37 = 1000  # Timeout
    # "User Events"
    n16 = call <vilib>:"Parse State Queue__jki_lib_state_machine.vi"("State Queue"=w43, "Error In (no error)"=w36) -> ("Remaining States"=w45:string, "Current State"=w32:string, "Arguments"=w44:string)  [unwired: 11 in]
    n17 = case shown="\"\", \"Event Structure\", \"Idle\"" w32 {
      selector: w32 -> [_ _ w584 _ _ _ _ _ _ _ _ _ _ _ _ _ _ _ _ _ _]
      tunnel: w45 -> [w60 w583 w588 w606 w612 w617 w621 w630 w639 w643 w652 w662 w673 w699 w704 w714 w718 w724 w733 w743 w752]
      tunnel: w44 -> [_ _ _ _ _ _ _ _ _ _ _ w657 w667 _ _ _ _ _ _ _ _]
      tunnel: w38 -> [w58 w580 w586 w597 w609 w615 w618 _ w634 w640 w650 w660 w669 w696 w701 w711 w715 w721 w727 w740 w747]
      tunnel: [w57 w581 w590 w603 errorcluster {"status"=FALSE, "code"=0, "source"=""} ("error out") w614 w619 w627 w635 w641 w645 w658 w670 w697 w702 w712 w716 w722 w731 w741 w750] -> w42
      tunnel: w36 -> [w56 w581 w589 w603 w608 w614 w619 w627 w636 w641 w649 w659 w671 w697 w702 w712 w716 w722 w731 w741 w750]
      tunnel: [w59 w582 w587 w605 w611 w616 w620 w629 w638 w642 w651 w661 w672 w698 w703 w713 w717 w723 w732 w742 w751] -> w41
      tunnel: [_ _ _ _ _ w613 _ _ _ _ _ _ _ _ _ _ _ _ _ _ _] -> w40
      tunnel: [w55 w580 w586 w604 w609 w615 w618 w626 w634 w640 w650 w660 w669 w696 w701 w711 w715 w721 w726 w740 w747] -> w39
      tunnel: w37 -> [w54 _ _ _ _ _ _ _ _ _ _ _ _ _ _ _ _ _ _ _ _]
      tunnel: w35 -> [w53 _ _ _ _ _ _ _ _ _ _ _ _ _ _ _ _ _ _ _ _]
      tunnel: w34 -> [w52 _ _ _ _ _ _ _ _ _ _ _ _ _ _ _ _ _ _ _ _]
      tunnel: w29 -> [w51 _ _ _ _ _ _ _ _ _ w647 _ _ _ _ _ _ _ _ _ _]
      tunnel: w28 -> [w50 _ _ _ _ _ _ _ _ _ _ _ _ _ _ _ _ _ _ _ _]
      frame "", "Event Structure", "Idle" {
        n18 = event shown="[39] \"Setup Test\": Value Change" {
          selector: _ -> [_ _ _ _ _ _ _ _ _ _ _ _ _ _ _ _ _ _ _ _ _ _ _ _ _ _ _ _ _ _ _ _ _ _ _ _ _ _ _ _ _ _ _]
          dyn-events: _ -> [_ _ _ _ _ _ _ _ _ _ _ _ _ _ _ _ _ _ _ _ _ _ _ _ _ _ _ _ _ _ _ _ _ _ _ _ _ _ _ _ _ _ _]
          timeout: w54 -> [_ _ _ _ _ _ _ _ _ _ _ _ _ _ _ _ _ _ _ _ _ _ _ _ _ _ _ _ _ _ _ _ _ _ _ _ _ _ _ _ _ _ _]
          tunnel: w60 -> [w65 w74 w84 w94 w104 w114 w124 w134 w144 w154 w164 w174 w184 w194 w204 w214 w224 w236 w248 w260 w273 w284 w296 w308 w321 w333 w347 w360 w373 w385 w399 w412 w424 w434 w443 w453 w461 w470 w481 w501 w525 w544 w579]
          tunnel: [w64 w74 w84 w94 w104 w114 w124 w134 w144 w154 w164 w174 w184 w194 w204 w214 w224 w236 w248 w260 w273 w284 w296 w308 w321 w332 w347 w360 w373 w385 w399 w412 w424 w434 w443 w453 w461 w470 w481 w501 w525 w544 w578] -> w59
          tunnel: w58 -> [w62 w75 w85 w95 w105 w115 w125 w135 w145 w155 w165 w175 w185 w195 w205 w215 w225 w237 w249 w261 w272 w285 w297 w309 w320 w335 w348 w361 w374 w386 w400 w413 w425 w435 w444 w452 w462 w469 w482 w486 w517 w536 w576]
          tunnel: [w63 w67 w78 w88 w98 w108 w118 w128 w137 w150 w159 w168 w177 w188 w198 w208 w218 w228 w243 w254 w265 w278 w290 w302 w314 w326 w339 w353 w366 w379 w392 w402 w418 w428 w437 w445 w454 w464 w475 w493 w520 w541 w577] -> w57
          tunnel: w56 -> [w63 w72 w79 w89 w99 w109 w119 w129 w138 w151 w160 w169 w179 w189 w199 w209 w219 w231 w244 w257 w267 w279 w291 w303 w313 w327 w340 w354 w367 w380 w393 w403 w419 w433 w440 w450 w460 w471 w476 w502 w524 w543 w577]
          tunnel: [w62 w75 w85 w95 w105 w115 w125 w135 w145 w155 w165 w175 w185 w195 w205 w215 w225 w237 w249 w261 w272 w285 w297 w309 w320 w335 w348 w361 w374 w386 w400 w413 w425 w435 w444 w452 w462 w469 w482 w485 w516 w535 w576] -> w55
          tunnel: w53 -> [_ _ _ _ _ _ _ _ _ _ _ _ _ _ _ _ _ _ _ _ _ _ _ _ _ _ _ _ _ _ _ _ _ _ _ _ _ _ _ _ _ w542 _]
          tunnel: w52 -> [_ _ _ _ _ _ _ _ _ _ _ _ _ _ _ _ _ _ _ _ _ _ _ _ _ _ _ _ _ _ _ _ _ _ _ _ _ _ _ w492 _ _ _]
          tunnel: w51 -> [_ w66 w76 w87 w96 w106 w116 w126 w136 w147 w157 w167 w176 w186 w196 w207 w217 w227 w242 w250 w268 w277 w289 w298 w315 w322 w341 w349 w362 w375 w388 w401 w414 w427 w436 w446 w455 _ _ _ _ _ _]
          tunnel: w50 -> [_ _ _ _ _ _ _ _ _ _ _ _ _ _ _ _ _ _ _ _ _ _ _ _ _ _ _ _ _ _ _ _ _ _ _ _ _ _ _ _ w519 _ _]
          event Timeout {
            n19 = event-data() -> ()  [unwired: 1 in, 1 out]
            n20 = call <vilib>:"Add State(s) to Queue__jki_lib_state_machine.vi"("State(s) in Front (\"\")"="Check Test Selected\nCheck Exit" ("State(s) in Front (\"\")"), "State(s) in (\"\")"=w65) -> ("States Out"=w64:string)  [unwired: 13 in]
          }
          event Value Change {
            n21 = event-data() -> ("NewVal"=w73:T23)  [unwired: 1 in, 5 out]
            n22 = call "RTS Ground Leak CMD.vi"("Station"=u16 1, "Error In"=w72, "NewVal in"=w73) -> ("Error Out"=w68:errorcluster, "Ground Leak CMD"=w70:string)  [unwired: 7 in]
            n23 = local write "Raw Command"(w70) -> ()
            n24 = Generate User Event(user event=w66, event data cluster=TRUE ("event data"), error in=w68) -> (error out=w67:errorcluster)  [unwired: 1 in, 1 out]
          }
          event Value Change {
            n25 = event-data() -> ("NewVal"=w77:T23)  [unwired: 1 in, 5 out]
            n26 = call "RTS Ground Leak CMD.vi"("Station"=u16 2, "Error In"=w79, "NewVal in"=w77) -> ("Error Out"=w80:errorcluster, "Ground Leak CMD"=w82:string)  [unwired: 7 in]
            n27 = local write "Raw Command"(w82) -> ()
            n28 = Generate User Event(user event=w76, event data cluster=TRUE ("event data"), error in=w80) -> (error out=w78:errorcluster)  [unwired: 1 in, 1 out]
          }
          event Value Change {
            n29 = event-data() -> ("NewVal"=w86:T23)  [unwired: 1 in, 5 out]
            n30 = call "RTS Ground Leak CMD.vi"("Station"=u16 3, "Error In"=w89, "NewVal in"=w86) -> ("Error Out"=w90:errorcluster, "Ground Leak CMD"=w92:string)  [unwired: 7 in]
            n31 = local write "Raw Command"(w92) -> ()
            n32 = Generate User Event(user event=w87, event data cluster=TRUE ("event data"), error in=w90) -> (error out=w88:errorcluster)  [unwired: 1 in, 1 out]
          }
          event Value Change {
            n33 = event-data() -> ("NewVal"=w97:T23)  [unwired: 1 in, 5 out]
            n34 = call "RTS Ground Leak CMD.vi"("Station"=u16 4, "Error In"=w99, "NewVal in"=w97) -> ("Error Out"=w100:errorcluster, "Ground Leak CMD"=w102:string)  [unwired: 7 in]
            n35 = local write "Raw Command"(w102) -> ()
            n36 = Generate User Event(user event=w96, event data cluster=TRUE ("event data"), error in=w100) -> (error out=w98:errorcluster)  [unwired: 1 in, 1 out]
          }
          event Value Change {
            n37 = event-data() -> ("NewVal"=w107:T23)  [unwired: 1 in, 5 out]
            n38 = call "RTS Ground Leak CMD.vi"("Station"=u16 5, "Error In"=w109, "NewVal in"=w107) -> ("Error Out"=w110:errorcluster, "Ground Leak CMD"=w112:string)  [unwired: 7 in]
            n39 = local write "Raw Command"(w112) -> ()
            n40 = Generate User Event(user event=w106, event data cluster=TRUE ("event data"), error in=w110) -> (error out=w108:errorcluster)  [unwired: 1 in, 1 out]
          }
          event Value Change {
            n41 = event-data() -> ("NewVal"=w117:T23)  [unwired: 1 in, 5 out]
            n42 = call "RTS Ground Leak CMD.vi"("Station"=u16 6, "Error In"=w119, "NewVal in"=w117) -> ("Error Out"=w120:errorcluster, "Ground Leak CMD"=w122:string)  [unwired: 7 in]
            n43 = local write "Raw Command"(w122) -> ()
            n44 = Generate User Event(user event=w116, event data cluster=TRUE ("event data"), error in=w120) -> (error out=w118:errorcluster)  [unwired: 1 in, 1 out]
          }
          event Value Change {
            n45 = event-data() -> ("NewVal"=w127:T23)  [unwired: 1 in, 5 out]
            n46 = call "RTS Ground Leak CMD.vi"("Station"=u16 7, "Error In"=w129, "NewVal in"=w127) -> ("Error Out"=w130:errorcluster, "Ground Leak CMD"=w132:string)  [unwired: 7 in]
            n47 = local write "Raw Command"(w132) -> ()
            n48 = Generate User Event(user event=w126, event data cluster=TRUE ("event data"), error in=w130) -> (error out=w128:errorcluster)  [unwired: 1 in, 1 out]
          }
          event Value Change {
            n49 = event-data() -> ("NewVal"=w139:T23)  [unwired: 1 in, 5 out]
            n50 = call "RTS Ground Leak CMD.vi"("Station"=u16 8, "Error In"=w138, "NewVal in"=w139) -> ("Error Out"=w140:errorcluster, "Ground Leak CMD"=w142:string)  [unwired: 7 in]
            n51 = local write "Raw Command"(w142) -> ()
            n52 = Generate User Event(user event=w136, event data cluster=TRUE ("event data"), error in=w140) -> (error out=w137:errorcluster)  [unwired: 1 in, 1 out]
          }
          event Value Change {
            n53 = event-data() -> ("NewVal"=w149:T21)  [unwired: 1 in, 5 out]
            n54 = call "RTS Polarity CMD.vi"("Station"=u16 1, "Error In"=w151, "NewVal"=w149) -> ("Error Out"=w153:errorcluster, "Polarity CMD"=w146:string)  [unwired: 7 in]
            n55 = local write "Raw Command"(w146) -> ()
            n56 = Generate User Event(user event=w147, event data cluster=TRUE ("event data"), error in=w153) -> (error out=w150:errorcluster)  [unwired: 1 in, 1 out]
          }
          event Value Change {
            n57 = event-data() -> ("NewVal"=w158:T21)  [unwired: 1 in, 5 out]
            n58 = call "RTS Polarity CMD.vi"("Station"=u16 2, "Error In"=w160, "NewVal"=w158) -> ("Error Out"=w163:errorcluster, "Polarity CMD"=w156:string)  [unwired: 7 in]
            n59 = local write "Raw Command"(w156) -> ()
            n60 = Generate User Event(user event=w157, event data cluster=TRUE ("event data"), error in=w163) -> (error out=w159:errorcluster)  [unwired: 1 in, 1 out]
          }
          event Value Change {
            n61 = event-data() -> ("NewVal"=w166:T21)  [unwired: 1 in, 5 out]
            n62 = call "RTS Polarity CMD.vi"("Station"=u16 3, "Error In"=w169, "NewVal"=w166) -> ("Error Out"=w172:errorcluster, "Polarity CMD"=w173:string)  [unwired: 7 in]
            n63 = local write "Raw Command"(w173) -> ()
            n64 = Generate User Event(user event=w167, event data cluster=TRUE ("event data"), error in=w172) -> (error out=w168:errorcluster)  [unwired: 1 in, 1 out]
          }
          event Value Change {
            n65 = event-data() -> ("NewVal"=w178:T21)  [unwired: 1 in, 5 out]
            n66 = call "RTS Polarity CMD.vi"("Station"=u16 4, "Error In"=w179, "NewVal"=w178) -> ("Error Out"=w182:errorcluster, "Polarity CMD"=w183:string)  [unwired: 7 in]
            n67 = local write "Raw Command"(w183) -> ()
            n68 = Generate User Event(user event=w176, event data cluster=TRUE ("event data"), error in=w182) -> (error out=w177:errorcluster)  [unwired: 1 in, 1 out]
          }
          event Value Change {
            n69 = event-data() -> ("NewVal"=w187:T21)  [unwired: 1 in, 5 out]
            n70 = call "RTS Polarity CMD.vi"("Station"=u16 5, "Error In"=w189, "NewVal"=w187) -> ("Error Out"=w192:errorcluster, "Polarity CMD"=w193:string)  [unwired: 7 in]
            n71 = local write "Raw Command"(w193) -> ()
            n72 = Generate User Event(user event=w186, event data cluster=TRUE ("event data"), error in=w192) -> (error out=w188:errorcluster)  [unwired: 1 in, 1 out]
          }
          event Value Change {
            n73 = event-data() -> ("NewVal"=w197:T21)  [unwired: 1 in, 5 out]
            n74 = call "RTS Polarity CMD.vi"("Station"=u16 6, "Error In"=w199, "NewVal"=w197) -> ("Error Out"=w202:errorcluster, "Polarity CMD"=w203:string)  [unwired: 7 in]
            n75 = local write "Raw Command"(w203) -> ()
            n76 = Generate User Event(user event=w196, event data cluster=TRUE ("event data"), error in=w202) -> (error out=w198:errorcluster)  [unwired: 1 in, 1 out]
          }
          event Value Change {
            n77 = event-data() -> ("NewVal"=w206:T21)  [unwired: 1 in, 5 out]
            n78 = call "RTS Polarity CMD.vi"("Station"=u16 7, "Error In"=w209, "NewVal"=w206) -> ("Error Out"=w212:errorcluster, "Polarity CMD"=w213:string)  [unwired: 7 in]
            n79 = local write "Raw Command"(w213) -> ()
            n80 = Generate User Event(user event=w207, event data cluster=TRUE ("event data"), error in=w212) -> (error out=w208:errorcluster)  [unwired: 1 in, 1 out]
          }
          event Value Change {
            n81 = event-data() -> ("NewVal"=w216:T21)  [unwired: 1 in, 5 out]
            n82 = call "RTS Polarity CMD.vi"("Station"=u16 8, "Error In"=w219, "NewVal"=w216) -> ("Error Out"=w222:errorcluster, "Polarity CMD"=w223:string)  [unwired: 7 in]
            n83 = local write "Raw Command"(w223) -> ()
            n84 = Generate User Event(user event=w217, event data cluster=TRUE ("event data"), error in=w222) -> (error out=w218:errorcluster)  [unwired: 1 in, 1 out]
          }
          event "Station Voltage Send 1": Value Change {
            n85 = event-data() -> ()  [unwired: 1 in, 6 out]
            n86 = call "RTS Client Volt Freq Command Send.vi"("Station"=u16 1, "Error In"=w231, "Voltage"="Voltage", "Frequency"="Frequency", "Wh Reset"="Wh Reset 1") -> ("Error Out"=w229:errorcluster, "Output Command"=→"Raw Command":string)  [unwired: 5 in]
            n87 = Generate User Event(user event=w227, event data cluster=TRUE ("event data"), error in=w229) -> (error out=w228:errorcluster)  [unwired: 1 in, 1 out]
          }
          event "Station Voltage Send 2": Value Change {
            n88 = event-data() -> ()  [unwired: 1 in, 6 out]
            n89 = call "RTS Client Volt Freq Command Send.vi"("Station"=u16 2, "Error In"=w244, "Voltage"="Voltage 2", "Frequency"="Frequency 2", "Wh Reset"="Wh Reset 2") -> ("Error Out"=w246:errorcluster, "Output Command"=w238:string)  [unwired: 5 in]
            n90 = local write "Raw Command"(w238) -> ()
            n91 = Generate User Event(user event=w242, event data cluster=TRUE ("event data"), error in=w246) -> (error out=w243:errorcluster)  [unwired: 1 in, 1 out]
          }
          event "Station Voltage Send 3": Value Change {
            n92 = event-data() -> ()  [unwired: 1 in, 6 out]
            n93 = call "RTS Client Volt Freq Command Send.vi"("Station"=u16 3, "Error In"=w257, "Voltage"="Voltage 3", "Frequency"="Frequency 3", "Wh Reset"="Wh Reset 3") -> ("Error Out"=w255:errorcluster, "Output Command"=w258:string)  [unwired: 5 in]
            n94 = local write "Raw Command"(w258) -> ()
            n95 = Generate User Event(user event=w250, event data cluster=TRUE ("event data"), error in=w255) -> (error out=w254:errorcluster)  [unwired: 1 in, 1 out]
          }
          event "Station Voltage Send 4": Value Change {
            n96 = event-data() -> ()  [unwired: 1 in, 6 out]
            n97 = call "RTS Client Volt Freq Command Send.vi"("Station"=u16 4, "Error In"=w267, "Voltage"="Voltage 4", "Frequency"="Frequency 4", "Wh Reset"="Wh Reset 4") -> ("Error Out"=w266:errorcluster, "Output Command"=w270:string)  [unwired: 5 in]
            n98 = local write "Raw Command"(w270) -> ()
            n99 = Generate User Event(user event=w268, event data cluster=TRUE ("event data"), error in=w266) -> (error out=w265:errorcluster)  [unwired: 1 in, 1 out]
          }
          event "Station Voltage Send 5": Value Change {
            n100 = event-data() -> ()  [unwired: 1 in, 6 out]
            n101 = call "RTS Client Volt Freq Command Send.vi"("Station"=u16 5, "Error In"=w279, "Voltage"="Voltage 5", "Frequency"="Frequency 5", "Wh Reset"="Wh Reset 5") -> ("Error Out"=w280:errorcluster, "Output Command"=w282:string)  [unwired: 5 in]
            n102 = local write "Raw Command"(w282) -> ()
            n103 = Generate User Event(user event=w277, event data cluster=TRUE ("event data"), error in=w280) -> (error out=w278:errorcluster)  [unwired: 1 in, 1 out]
          }
          event "Station Voltage Send 6": Value Change {
            n104 = event-data() -> ()  [unwired: 1 in, 6 out]
            n105 = call "RTS Client Volt Freq Command Send.vi"("Station"=u16 6, "Error In"=w291, "Voltage"="Voltage 6", "Frequency"="Frequency 6", "Wh Reset"="Wh Reset 6") -> ("Error Out"=w292:errorcluster, "Output Command"=w294:string)  [unwired: 5 in]
            n106 = local write "Raw Command"(w294) -> ()
            n107 = Generate User Event(user event=w289, event data cluster=TRUE ("event data"), error in=w292) -> (error out=w290:errorcluster)  [unwired: 1 in, 1 out]
          }
          event "Station Voltage Send 7": Value Change {
            n108 = event-data() -> ()  [unwired: 1 in, 6 out]
            n109 = call "RTS Client Volt Freq Command Send.vi"("Station"=u16 7, "Error In"=w303, "Voltage"="Voltage 7", "Frequency"="Frequency 7", "Wh Reset"="Wh Reset 7") -> ("Error Out"=w304:errorcluster, "Output Command"=w306:string)  [unwired: 5 in]
            n110 = local write "Raw Command"(w306) -> ()
            n111 = Generate User Event(user event=w298, event data cluster=TRUE ("event data"), error in=w304) -> (error out=w302:errorcluster)  [unwired: 1 in, 1 out]
          }
          event "Station Voltage Send 8": Value Change {
            n112 = event-data() -> ()  [unwired: 1 in, 6 out]
            n113 = call "RTS Client Volt Freq Command Send.vi"("Station"=u16 8, "Error In"=w313, "Voltage"="Voltage 8", "Frequency"="Frequency 8", "Wh Reset"="Wh Reset 8") -> ("Error Out"=w316:errorcluster, "Output Command"=w318:string)  [unwired: 5 in]
            n114 = local write "Raw Command"(w318) -> ()
            n115 = Generate User Event(user event=w315, event data cluster=TRUE ("event data"), error in=w316) -> (error out=w314:errorcluster)  [unwired: 1 in, 1 out]
          }
          event "Station 1 CMD": Value Change {
            n116 = event-data() -> ()  [unwired: 1 in, 6 out]
            n117 = Unbundle By Name("Door Settings") -> ("Station 1.Slide"=w323:T28, "Station 1.Cab"=w324:T28, "Station 1.Freezer"=w325:T28)
            n118 = call "RTS Door CMD.vi"("Station"=u16 1, "Error In"=w327, "Freezer"=w325, "Cab"=w324, "Slide"=w323) -> ("Error Out"=w329:errorcluster, "Door CMD"=w331:string)  [unwired: 5 in]
            n119 = Generate User Event(user event=w322, event data cluster=TRUE ("event data"), error in=w329) -> (error out=w326:errorcluster)  [unwired: 1 in, 1 out]
            n120 = local write "Raw Command"(w331) -> ()
            n121 = call <vilib>:"Add State(s) to Queue__jki_lib_state_machine.vi"("State(s) in (\"\")"=w333) -> ("States Out"=w332:string)  [unwired: 14 in]
          }
          event "Station 2 CMD": Value Change {
            n122 = event-data() -> ()  [unwired: 1 in, 6 out]
            n123 = local read "Door Settings"() -> (w346:T26)
            n124 = Unbundle By Name(w346) -> ("Station 2.Slide"=w338:T28, "Station 2.Cab"=w337:T28, "Station 2.Freezer"=w336:T28)
            n125 = call "RTS Door CMD.vi"("Station"=u16 2, "Error In"=w340, "Freezer"=w336, "Cab"=w337, "Slide"=w338) -> ("Error Out"=w343:errorcluster, "Door CMD"=w345:string)  [unwired: 5 in]
            n126 = Generate User Event(user event=w341, event data cluster=TRUE ("event data"), error in=w343) -> (error out=w339:errorcluster)  [unwired: 1 in, 1 out]
            n127 = local write "Raw Command"(w345) -> ()
          }
          event "Station 3 CMD": Value Change {
            n128 = event-data() -> ()  [unwired: 1 in, 6 out]
            n129 = local read "Door Settings"() -> (w359:T26)
            n130 = Unbundle By Name(w359) -> ("Station 3.Slide"=w350:T28, "Station 3.Cab"=w351:T28, "Station 3.Freezer"=w352:T28)
            n131 = call "RTS Door CMD.vi"("Station"=u16 3, "Error In"=w354, "Freezer"=w352, "Cab"=w351, "Slide"=w350) -> ("Error Out"=w356:errorcluster, "Door CMD"=w358:string)  [unwired: 5 in]
            n132 = Generate User Event(user event=w349, event data cluster=TRUE ("event data"), error in=w356) -> (error out=w353:errorcluster)  [unwired: 1 in, 1 out]
            n133 = local write "Raw Command"(w358) -> ()
          }
          event "Station 4 CMD": Value Change {
            n134 = event-data() -> ()  [unwired: 1 in, 6 out]
            n135 = local read "Door Settings"() -> (w372:T26)
            n136 = Unbundle By Name(w372) -> ("Station 4.Slide"=w363:T28, "Station 4.Cab"=w364:T28, "Station 4.Freezer"=w365:T28)
            n137 = call "RTS Door CMD.vi"("Station"=u16 4, "Error In"=w367, "Freezer"=w365, "Cab"=w364, "Slide"=w363) -> ("Error Out"=w369:errorcluster, "Door CMD"=w371:string)  [unwired: 5 in]
            n138 = Generate User Event(user event=w362, event data cluster=TRUE ("event data"), error in=w369) -> (error out=w366:errorcluster)  [unwired: 1 in, 1 out]
            n139 = local write "Raw Command"(w371) -> ()
          }
          event "Station 5 CMD": Value Change {
            n140 = event-data() -> ()  [unwired: 1 in, 6 out]
            n141 = local read "Door Settings"() -> (w387:T26)
            n142 = Unbundle By Name(w387) -> ("Station 5.Slide"=w376:T28, "Station 5.Cab"=w377:T28, "Station 5.Freezer"=w378:T28)
            n143 = call "RTS Door CMD.vi"("Station"=u16 5, "Error In"=w380, "Freezer"=w378, "Cab"=w377, "Slide"=w376) -> ("Error Out"=w382:errorcluster, "Door CMD"=w384:string)  [unwired: 5 in]
            n144 = Generate User Event(user event=w375, event data cluster=TRUE ("event data"), error in=w382) -> (error out=w379:errorcluster)  [unwired: 1 in, 1 out]
            n145 = local write "Raw Command"(w384) -> ()
          }
          event "Station 6 CMD": Value Change {
            n146 = event-data() -> ()  [unwired: 1 in, 6 out]
            n147 = local read "Door Settings"() -> (w398:T26)
            n148 = Unbundle By Name(w398) -> ("Station 6.Slide"=w389:T28, "Station 6.Cab"=w390:T28, "Station 6.Freezer"=w391:T28)
            n149 = call "RTS Door CMD.vi"("Station"=u16 6, "Error In"=w393, "Freezer"=w391, "Cab"=w390, "Slide"=w389) -> ("Error Out"=w395:errorcluster, "Door CMD"=w397:string)  [unwired: 5 in]
            n150 = Generate User Event(user event=w388, event data cluster=TRUE ("event data"), error in=w395) -> (error out=w392:errorcluster)  [unwired: 1 in, 1 out]
            n151 = local write "Raw Command"(w397) -> ()
          }
          event "Station 7 CMD": Value Change {
            n152 = event-data() -> ()  [unwired: 1 in, 6 out]
            n153 = local read "Door Settings"() -> (w411:T26)
            n154 = Unbundle By Name(w411) -> ("Station 7.Slide"=w404:T28, "Station 7.Cab"=w405:T28, "Station 7.Freezer"=w406:T28)
            n155 = call "RTS Door CMD.vi"("Station"=u16 7, "Error In"=w403, "Freezer"=w406, "Cab"=w405, "Slide"=w404) -> ("Error Out"=w408:errorcluster, "Door CMD"=w410:string)  [unwired: 5 in]
            n156 = Generate User Event(user event=w401, event data cluster=TRUE ("event data"), error in=w408) -> (error out=w402:errorcluster)  [unwired: 1 in, 1 out]
            n157 = local write "Raw Command"(w410) -> ()
          }
          event "Station 8 CMD": Value Change {
            n158 = event-data() -> ()  [unwired: 1 in, 6 out]
            n159 = local read "Door Settings"() -> (w426:T26)
            n160 = Unbundle By Name(w426) -> ("Station 8.Slide"=w415:T28, "Station 8.Cab"=w416:T28, "Station 8.Freezer"=w417:T28)
            n161 = call "RTS Door CMD.vi"("Station"=u16 8, "Error In"=w419, "Freezer"=w417, "Cab"=w416, "Slide"=w415) -> ("Error Out"=w421:errorcluster, "Door CMD"=w423:string)  [unwired: 5 in]
            n162 = local write "Raw Command"(w423) -> ()
            n163 = Generate User Event(user event=w414, event data cluster=TRUE ("event data"), error in=w421) -> (error out=w418:errorcluster)  [unwired: 1 in, 1 out]
          }
          event Value Change {
            # "Enable the Door Openers"
            n164 = event-data() -> ("NewVal"=w432:T29)  [unwired: 1 in, 5 out]
            n165 = call "RTS Enable Door CMD.vi"("Error In"=w433, "Enable Door"=w432) -> ("Error Out"=w429:errorcluster, "Door CMD"=w431:string)  [unwired: 8 in]
            n166 = local write "Raw Command"(w431) -> ()
            n167 = Generate User Event(user event=w427, event data cluster=TRUE ("event data"), error in=w429) -> (error out=w428:errorcluster)  [unwired: 1 in, 1 out]
          }
          event Value Change {
            n168 = event-data() -> ("NewVal"=w441:T4)  [unwired: 1 in, 5 out]
            n169 = call "RTS Room OK CMD.vi"("Error In"=w440, "Room OK?"=w441) -> ("Error Out"=w438:errorcluster, "Room OK CMD"=w442:string)  [unwired: 8 in]
            n170 = local write "Raw Command"(w442) -> ()
            n171 = Generate User Event(user event=w436, event data cluster=TRUE ("event data"), error in=w438) -> (error out=w437:errorcluster)  [unwired: 1 in, 1 out]
          }
          event Value Change {
            n172 = event-data() -> ("NewVal"=w449:T5)  [unwired: 1 in, 5 out]
            n173 = call "RTS Room Run CMD.vi"("Error In"=w450, "Room Run"=w449) -> ("Error Out"=w447:errorcluster, "Room OK CMD"=w451:string)  [unwired: 8 in]
            n174 = local write "Raw Command"(w451) -> ()
            n175 = Generate User Event(user event=w446, event data cluster=TRUE ("event data"), error in=w447) -> (error out=w445:errorcluster)  [unwired: 1 in, 1 out]
          }
          event "Update Room Setpoint": Value Change {
            n176 = event-data() -> ()  [unwired: 1 in, 6 out]
            n177 = call "RTS Chamber Control CMD.vi"("Error In"=w460, "Room Setpoints"="Room Setpoints") -> ("Error Out"=w456:errorcluster, "Output Command"=w459:string)  [unwired: 8 in]
            n178 = local write "Raw Command"(w459) -> ()
            n179 = Generate User Event(user event=w455, event data cluster=TRUE ("event data"), error in=w456) -> (error out=w454:errorcluster)  [unwired: 1 in, 1 out]
          }
          event Value Change {
            n180 = event-data() -> ("NewVal"=w466:dbl)  [unwired: 1 in, 5 out]
            n181 = local read "Room Setpoints"() -> (w467:T30)
            n182 = Bundle By Name(cluster=w467, "Room Setpoint Temperature (*RM Dry Set P1)"=w466) -> (w468:T30)
            n183 = call "RTS Calculate Chamber CoolDehum Temps.vi"("Error In"=w471, "Room Setpoints"=w468) -> ("Error Out"=w465:errorcluster, "Room Setpoint Output"=w463:T30)  [unwired: 8 in]
            n184 = flat-sequence {
              tunnel: w465 -> [w473]
              tunnel: [w473] -> w464
              tunnel: w463 -> [w472]
              frame #0 {
                n185 = local write "Room Setpoints"(w472) -> ()
              }
            }
          }
          event Value Change {
            n186 = event-data() -> ("NewVal"=w474:dbl)  [unwired: 1 in, 5 out]
            n187 = local read "Room Setpoints"() -> (w479:T30)
            n188 = Bundle By Name(cluster=w479, "Room Setpoint Humidity (*RM Hum Set P1)"=w474) -> (w480:T30)
            n189 = call "RTS Calculate Chamber CoolDehum Temps.vi"("Error In"=w476, "Room Setpoints"=w480) -> ("Error Out"=w478:errorcluster, "Room Setpoint Output"=w477:T30)  [unwired: 8 in]
            n190 = flat-sequence {
              tunnel: w478 -> [w484]
              tunnel: [w484] -> w475
              tunnel: w477 -> [w483]
              frame #0 {
                n191 = local write "Room Setpoints"(w483) -> ()
              }
            }
          }
          event "Setup Test": Value Change {
            n192 = event-data() -> ()  [unwired: 1 in, 6 out]
            n193 = local read "Tree Selection"() -> (w487:T1)
            n194 = Unbundle By Name(w486) -> ("Filepath"=w495:T2)
            n195 = call "Save File DOE File Setup.vi"("Filepath In"=w495, "Station ID:"=w487, "error in (no error)"=w502, "Config State"=Save_File_DOE_Configuration_State."Open Front Panel", "LV Program"=Save_File_DOE_LabView_Program."Refrigeration") -> ("Washer Controls Out"=w499:T39, "Filepath Out"=w503:T2, "error out"=w494:errorcluster)  [unwired: 12 in]
            n196 = Unbundle By Name(w499) -> ("Initialize.Washer In.Appliance Details.File Name Output Array"=w498:string[][])
            n197 = Unbundle By Name(w503) -> ("Data File Paths.Data File Path"=w488:path)
            n198 = Array To Spreadsheet String(delimiter (Tab)=",", array=w498, 3:"%s" ("format string")) -> (spreadsheet string=w489:string)
            n199 = String Length(string=w489) -> (length=w491:i32)
            n200 = Greater Than 0?(x=w491) -> (x > 0?=w490:bool)
            n201 = case shown="True" w490 {
              tunnel: w492 -> [_ w515]
              tunnel: w494 -> [w506 w514]
              tunnel: [w506 w513] -> w493
              tunnel: w489 -> [_ w511]
              tunnel: w488 -> [_ w510]
              tunnel: w486 -> [w505 w509]
              tunnel: [w505 w508] -> w485
              frame False {
              }
              frame True {
                n202 = Bundle By Name(cluster=w509, "File Name Selected?"=TRUE) -> (w508:T61)
                n203 = Generate User Event(user event=w515, event data cluster=TRUE ("event data"), error in=w514) -> (error out=w513:errorcluster)  [unwired: 1 in, 1 out]
                "Setup Info" <- w511
                "Data File Path" <- w510
              }
            }
          }
          event "Test Setup": Value Change {
            n204 = event-data() -> ()  [unwired: 1 in, 6 out]
            n205 = local read "RTS Config Setup Output"() -> (w523:T6)
            n206 = Unbundle By Name(w523) -> ("Station Settings"=w522:T12)
            n207 = call "RTS Door Opener Setup.vi"("Error In"=w524, "Station Settings"=w522) -> ("Error Out"=w521:errorcluster, "Update Server Output"=w518:bool)  [unwired: 8 in]
            n208 = case shown="True" w518 {
              tunnel: w519 -> [_ w534]
              tunnel: w521 -> [w527 w533]
              tunnel: [w527 w532] -> w520
              tunnel: w517 -> [w526 w529]
              tunnel: [w526 w528] -> w516
              frame False {
              }
              frame True {
                n209 = Generate User Event(user event=w534, event data cluster=TRUE ("event data"), error in=w533) -> (error out=w532:errorcluster)  [unwired: 1 in, 1 out]
                n210 = Bundle By Name(cluster=w529, "Test Selected?"=TRUE ("Point File Selected?")) -> (w528:T61)
              }
            }
          }
          event "Configure Point File": Value Change {
            n211 = event-data() -> ()  [unwired: 1 in, 6 out]
            n212 = Unbundle By Name(w536) -> ("Filepath.General Setup Paths.General Startup Config Path"=w537:path)
            n213 = local read "Tree Selection"() -> (w539:T1)
            n214 = Equal?(x=w539, y="Select Room/Stall") -> (x = y?=w540:bool)
            n215 = case shown="False" w540 {
              tunnel: w543 -> [w556 w573]
              tunnel: w542 -> [w555 _]
              tunnel: [w553 w573] -> w541
              tunnel: w539 -> [w549 _]
              tunnel: w537 -> [w547 _]
              tunnel: w536 -> [w546 w571]
              tunnel: [w545 w571] -> w535
              frame False {
                n216 = local read "Chamber Data"() -> (w550:string[][])
                n217 = call "Dynamic Headers Change Headers.vi"("Tree Selection"=w549, "Error In"=w556, "Tool Base Path"=w547, "Chamber Data"=w550) -> ("Error Out"=w554:errorcluster, "Point File Path"=w551:path, "Default Headers"=w548:bool)  [unwired: 4 in, 1 out]
                n218 = case shown="False" w548 {
                  tunnel: [w558 FALSE] -> w552
                  tunnel: w551 -> [w557 _]
                  frame False {
                    n219 = Equal?(x=w557, y=path "") -> (x = y?=w558:bool)
                  }
                  frame True {
                  }
                }
                n220 = case shown="False" w552 {
                  tunnel: w555 -> [w568 _]
                  tunnel: w554 -> [w567 w570]
                  tunnel: [w566 w570] -> w553
                  tunnel: w551 -> [w564 _]
                  tunnel: w549 -> [_ _]
                  tunnel: w546 -> [w563 w569]
                  tunnel: [w562 w569] -> w545
                  frame False {
                    n221 = Bundle By Name(cluster=w563, "Point File Selected?"=TRUE) -> (w562:T61)
                    n222 = Generate User Event(user event=w568, event data cluster=TRUE ("event data"), error in=w567) -> (error out=w566:errorcluster)  [unwired: 1 in, 1 out]
                    "Point File Path" <- w564
                  }
                  frame True {
                  }
                }
              }
              frame True {
                n223 = One Button Dialog(message="Select Station to Configure") -> ()  [unwired: 1 in, 1 out]
              }
            }
          }
          event Panel Close? {
            # "Discard the event because we'll close the front panel ourselves in Macro: Exit"
            # "Close Panel button (pressed) Event\n(this executes Macro: Exit to terminate the VI)"
            n224 = event-data() -> ()  [unwired: 1 in, 1 out]
            n225 = call <vilib>:"Add State(s) to Queue__jki_lib_state_machine.vi"("State(s) in Front (\"\")"="Macro: Exit", "State(s) in (\"\")"=w579) -> ("States Out"=w578:string)  [unwired: 13 in]
            n226 = event-data("Discard?"=TRUE) -> ()  [unwired: 1 in, 1 out]
          }
        }
      }
      frame "---------- Core ----------" {
        # "Do not put any code in this frame.\n(it is a separator no-op)"
        n227 = call <vilib>:"Add State(s) to Queue__jki_lib_state_machine.vi"("State(s) in (\"\")"=w583) -> ("States Out"=w582:string)  [unwired: 14 in]
      }
      frame Default {
        w593 = 42 items=["No error", "Argument error", "Memory is full", "Out of zone", "End of file", "File already open", "Generic file I/O error", "File not found", "File permission error", "Disk is full", "Duplicate path", "Too many files open", "System feature not enabled", "Resource file not found", "Cannot add resource", "Resource not found", "Image not found", "Image memory error", "Pen does not exist", "Config type invalid", "Config token not found", "Config parse error", "Config memory error", "Bad external code format", "Bad external code offset", "External code not present", "Null window", "Destroy window error", "Null menu", "Print aborted", "Bad print record", "Print driver error", "Windows error during printing", "Memory error during printing", "Print dialog error", "Generic print error", "Invalid device refnum", "Device not found", "Device parameter error", "Device unit error", "Cannot open device", "Device call aborted", "Generic error", "Cancelled by user", "Object ID too low", "Object ID too high", "Object not in heap", "Unknown heap", "Unknown object (invalid DefProc)", "Unknown object (DefProc not in table)", "Message out of range", "Invalid (null) method", "Unknown message", "Manager call not supported", "Bad address", "Network operation in progress", "Network operation timed out", "Connection is busy", "Network attribute not supported", "Network error", "Address in use", "System out of memory", "Connection aborted", "Connection refused", "Not connected", "Already connected", "Connection closed", "Initialization error (interapplication manager)", "Bad occurrence", "Wait on unbound occurrence handler", "Occurrence queue overflow", "Datalog type conflict", "Unused", "Unrecognized type (interapplication manager)", "Memory corrupt", "Failed to make temporary DLL", "Old CIN version", "Drag socket not found", "Failed to load drop-object", "Failed to register OLE object", "Failed to release OLE object", "Format specifier type mismatch", "Unknown format specifier", "Too few format specifiers", "Too many format specifiers", "Scan failed", "Newer CIN version", "Error converting to variant", "Runtime menu error", "Password tampered", "Variant attribute not found", "Incompatible variant data type", "Event data is not available", "Event Store is not present", "Occurrence is not found", "Event Queue is not created", "Event info is not available", "Refnum passed is NULL", "Error retrieving Class GUID", "Error retrieving CoClass GUID", "Error retrieving TypeLib GUID.", "Bad built application magic bytes.", "Specific driver is different from the specific driver associated with the Logical Name.", "There is no session opened to the class driver.", "Max Error", "MAX - Error with config objects", "MAX - Error loading configuration", "MAX - Group not supported"]
        # "Current State"
        # "Do not delete, rename, or modify this frame.\n(this is used to capture unhandled states and typos)"
        # "Handle mistyped state name (developer tool)"
        n228 = Format Into String(format string="Software Exception: Unhandled State \"%s\"." ("message"), error in=w589, w584) -> (resulting string=w592:string, error out=w591:errorcluster)  [unwired: 1 in]
        n229 = call <vilib>:"Error Cluster From Error Code.vi"("show call chain? (False)"=TRUE, "error in (no error)"=w591, "error message (\"\")"=w592, "error code (0)"=w593) -> ("error out"=w590:errorcluster)  [unwired: 5 in]
        n230 = call <vilib>:"Add State(s) to Queue__jki_lib_state_machine.vi"("State(s) in (\"\")"=w588) -> ("States Out"=w587:string)  [unwired: 14 in]
      }
      frame "Initialize Core Data" {
        # "Do not delete, rename, or modify this frame.\n(this is used to determine panel behavior on exit)"
        # "originally closed?"
        # "exe?"
        # "If panel starts closed or is an EXE, then close it when we exit"
        n231 = property class="VI"() -> ("Front Panel.Open"=w602:bool)  [unwired: 2 in, 2 out]
        n232 = property class="App"() -> ("App.Kind"=w601:T37)  [unwired: 2 in, 2 out]
        n233 = control-ref of="Current VI Reference"() -> (w595:refnum<vi>)
        n234 = Not(x=w602) -> (.not. x?=w599:bool)
        n235 = Equal?(x=w601, y=T37."Run Time System" ("Application:Kind")) -> (x = y?=w598:bool)
        n236 = Or(x=w599, y=w598) -> (x .or. y?=w596:bool)
        n237 = Bundle By Name(cluster=w597, "Core.Current VI Reference"=w595, "Core.Close Panel on Exit?"=w596) -> (w604:T61)
        n238 = call <vilib>:"Add State(s) to Queue__jki_lib_state_machine.vi"("State(s) in (\"\")"=w606) -> ("States Out"=w605:string)  [unwired: 14 in]
      }
      frame "Error Handler" {
        # "Unhandled Error -- Display it"
        # "Handle any errors here.\nYou can also output any states to clean-up after errors occur"
        # "Clear error"
        n239 = call <vilib>:"General Error Handler.vi"("error in (no error)"=w608) -> ()  [unwired: 10 in, 5 out]
        n240 = call <vilib>:"Add State(s) to Queue__jki_lib_state_machine.vi"("State(s) in Front (\"\")"="/* Post Error States", "State(s) in (\"\")"=w612) -> ("States Out"=w611:string)  [unwired: 13 in]
      }
      frame "Exit" {
        w613 = TRUE
        # "Do not put any code in this frame.\n(No errors that occur here will be handled.)"
        n241 = call <vilib>:"Add State(s) to Queue__jki_lib_state_machine.vi"("State(s) in (\"\")"=w617) -> ("States Out"=w616:string)  [unwired: 14 in]
        "System Exit" <- w613
      }
      frame "---------- Data ----------" {
        n242 = call <vilib>:"Add State(s) to Queue__jki_lib_state_machine.vi"("State(s) in (\"\")"=w621) -> ("States Out"=w620:string)  [unwired: 14 in]
      }
      frame "Data: Initialize" {
        w622 = FALSE  # File Name Selected?
        w623 = FALSE  # Point File Selected?
        w624 = FALSE  # Test Selected?
        w628 = T62 {"Current VI Reference"=refnum, "Close Panel on Exit?"=FALSE}  # Core
        n243 = while {
          tunnel: [w631] -> w625
          stop <- w633 stop-if-true
          n244 = Wait Until Next ms Multiple(millisecond multiple=u32 100) -> ()  [unwired: 1 out]
          n245 = local read "Start UI Loop"() -> (w633:bool)
          n246 = local read "Filepath"() -> (w631:T2)
        }
        n247 = call <vilib>:"Add State(s) to Queue__jki_lib_state_machine.vi"("State(s) in (\"\")"=w630) -> ("States Out"=w629:string)  [unwired: 14 in]
        n248 = Bundle("Core"=w628, "Filepath"=w625, "Test Selected?"=w624, "Point File Selected?"=w623, "File Name Selected?"=w622) -> (w626:T61)  [unwired: 1 in]
      }
      frame "Data: Cleanup" {
        # "Cleanup any data and references, here.\n(this is called automatically, by the Macro: Exit)"
        n249 = Unbundle By Name(w634) -> ("Core.Current VI Reference"=w637:refnum<vi>)
        n250 = Close Reference(reference=w637, error in (no error)=w636) -> (error out=w635:errorcluster)
        n251 = call <vilib>:"Add State(s) to Queue__jki_lib_state_machine.vi"("State(s) in (\"\")"=w639) -> ("States Out"=w638:string)  [unwired: 14 in]
      }
      frame "---------- UI ----------" {
        # "Do not put any code in this frame.\n(It is a separator no-op. You can make a copy of this frame to create a new UI frame)"
        n252 = call <vilib>:"Add State(s) to Queue__jki_lib_state_machine.vi"("State(s) in (\"\")"=w643) -> ("States Out"=w642:string)  [unwired: 14 in]
      }
      frame "UI: Initialize" {
        n253 = flat-sequence {
          tunnel: w649 -> [w653]
          tunnel: [w653] -> w644
          tunnel: [w656] -> w646
          tunnel: w644 -> [w656]
          frame #0 {
            n254 = property on="Tree Selection" class="CmbBox (strict)"("DisabledEnum"=T34."Enabled" ("Disabled")) -> ()  [unwired: 2 in, 2 out]
          }
          frame #1 {
            # "Get setup data from server"
            n255 = local write "Raw Command"(T33 "Get Setup" ("TCP Commands")) -> ()
          }
        }
        n256 = call <vilib>:"Add State(s) to Queue__jki_lib_state_machine.vi"("State(s) in (\"\")"=w652) -> ("States Out"=w651:string)  [unwired: 14 in]
        n257 = Generate User Event(user event=w647, event data cluster=TRUE ("event data"), error in=w646) -> (error out=w645:errorcluster)  [unwired: 1 in, 1 out]
      }
      frame "UI: Cursor Set" {
        # "Argument"
        # "Set and Unset Cursor Busy.\n(Usage: \"UI: Cursor Set >> Busy|Idle\")"
        n258 = case shown="\"Idle\", Default" w657 {
          tunnel: w659 -> [w664 w666]
          tunnel: [w663 w665] -> w658
          frame "Idle", Default {
            n259 = call <vilib>:"Unset Busy.vi"("error in (no error)"=w664) -> ("error out"=w663:errorcluster)  [unwired: 10 in]
          }
          frame "Busy" {
            n260 = call <vilib>:"Set Busy.vi"("error in (no error)"=w666) -> ("error out"=w665:errorcluster)  [unwired: 9 in, 1 out]
          }
        }
        n261 = call <vilib>:"Add State(s) to Queue__jki_lib_state_machine.vi"("State(s) in (\"\")"=w662) -> ("States Out"=w661:string)  [unwired: 14 in]
      }
      frame "UI: Front Panel State" {
        # "Argument"
        # "Set Front Panel Open or Closed\n(Usage: \"UI: Front Panel State >> Open|Close\")"
        n262 = Unbundle By Name(w669) -> ("Core.Current VI Reference"=w668:refnum<vi>)
        n263 = case shown="\"Open\", Default" w667 {
          tunnel: w671 -> [w677 w690]
          tunnel: [w679 w691] -> w670
          tunnel: w668 -> [w678 w688]
          frame "Open", Default {
            n264 = property class="VI"(reference=w678, error in=w677) -> (reference out=w675:refnum<vi>, error out=w676:errorcluster, "Front Panel.Open"=w674:bool)
            n265 = case shown="False" w674 {
              tunnel: [w682 w685] -> w679
              tunnel: w676 -> [w681 w685]
              tunnel: w675 -> [w680 _]
              frame False {
                n266 = invoke class="VI" method="FP.Open"(reference=w680, error in=w681, "Activate"=TRUE, "State"=T38."Standard") -> (error out=w682:errorcluster)  [unwired: 1 in, 4 out]
              }
              frame True {
              }
            }
          }
          frame "Close" {
            n267 = property class="VI"(reference=w688, error in=w690) -> (reference out=w687:refnum<vi>, error out=w689:errorcluster, "Front Panel.Open"=w686:bool)
            n268 = case shown="True" w686 {
              tunnel: [w692 w695] -> w691
              tunnel: w689 -> [w692 w694]
              tunnel: w687 -> [_ w693]
              frame False {
              }
              frame True {
                n269 = invoke class="VI" method="FP.Close"(reference=w693, error in=w694) -> (error out=w695:errorcluster)  [unwired: 1 in, 2 out]
              }
            }
          }
        }
        n270 = call <vilib>:"Add State(s) to Queue__jki_lib_state_machine.vi"("State(s) in (\"\")"=w673) -> ("States Out"=w672:string)  [unwired: 14 in]
      }
      frame "---------- Macro ----------" {
        # "Do not put any code in this frame.\n(It is a separator no-op. You can make a copy of this frame to create a new Macro frame)"
        n271 = call <vilib>:"Add State(s) to Queue__jki_lib_state_machine.vi"("State(s) in (\"\")"=w699) -> ("States Out"=w698:string)  [unwired: 14 in]
      }
      frame "Macro: Initialize" {
        w700 = "Data: Initialize\nInitialize Core Data\nUI: Initialize\nUI: Front Panel State >> Open"  # Data: Initialize Initialize Core Data UI: Initialize UI: Front Panel State >> Open
        n272 = call <vilib>:"Add State(s) to Queue__jki_lib_state_machine.vi"("State(s) in Front (\"\")"=w700, "State(s) in (\"\")"=w704) -> ("States Out"=w703:string)  [unwired: 13 in]
      }
      frame "Macro: Exit" {
        # "Exit Macro\n(This is called once, when the VI exits)"
        n273 = Unbundle By Name(w711) -> ("Core.Close Panel on Exit?"=w710:bool)
        n274 = Select(t="UI: Front Panel State >> Close", s=w710, f="") -> (s? t:f=w707:string)
        n275 = call <vilib>:"Add State(s) to Queue__jki_lib_state_machine.vi"("State(s) in (\"\")"=w707, "State(s) at Back (\"\")"="Data: Cleanup\nExit") -> ("States Out"=w705:string)  [unwired: 13 in]
        n276 = call <vilib>:"Add State(s) to Queue__jki_lib_state_machine.vi"("State(s) in Front (\"\")"=w705, "State(s) in (\"\")"=w714) -> ("States Out"=w713:string)  [unwired: 13 in]
      }
      frame "---------- New Category ----------" {
        # "Template Separator\n(You can make a copy of, or modify, this frame)"
        n277 = call <vilib>:"Add State(s) to Queue__jki_lib_state_machine.vi"("State(s) in (\"\")"=w718) -> ("States Out"=w717:string)  [unwired: 14 in]
      }
      frame "Check Test Selected" {
        n278 = local read "Tree Selection"() -> (w720:T1)
        n279 = local read "RTS Config Setup Output"() -> (w719:T6)
        n280 = case shown="\"1-1\"" w720 {
          tunnel: w719 -> [_ w725 _ _ _ _ _ _ _ _ _ _ _ _ _ _ _ _ _ _ _ _ _ _ _ _ _ _ _ _ _ _ _]
          frame "Select Room/Stall", Default {
          }
          frame "1-1" {
            n281 = Unbundle By Name(w725) -> ()  [unwired: 1 out]
          }
          frame "1-2" {
          }
          frame "1-3" {
          }
          frame "1-4" {
          }
          frame "1-5" {
          }
          frame "1-6" {
          }
          frame "1-7" {
          }
          frame "1-8" {
          }
          frame "2-1" {
          }
          frame "2-2" {
          }
          frame "2-3" {
          }
          frame "2-4" {
          }
          frame "2-5" {
          }
          frame "2-6" {
          }
          frame "2-7" {
          }
          frame "2-8" {
          }
          frame "3-1" {
          }
          frame "3-2" {
          }
          frame "3-3" {
          }
          frame "3-4" {
          }
          frame "3-5" {
          }
          frame "3-6" {
          }
          frame "3-7" {
          }
          frame "3-8" {
          }
          frame "4-1" {
          }
          frame "4-2" {
          }
          frame "4-3" {
          }
          frame "4-4" {
          }
          frame "4-5" {
          }
          frame "4-6" {
          }
          frame "4-7" {
          }
          frame "4-8" {
          }
        }
        n282 = call <vilib>:"Add State(s) to Queue__jki_lib_state_machine.vi"("State(s) in (\"\")"=w724) -> ("States Out"=w723:string)  [unwired: 14 in]
      }
      frame "Check Point File" {
        n283 = property on="Configure Point File" class="Bool"() -> ("BoolText.Text"=w730:string)  [unwired: 2 in, 2 out]
        n284 = Equal?(x=w730, y="Configure Point File") -> (x = y?=w728:bool)
        n285 = case shown="False" w728 {
          tunnel: w727 -> [w735 w739]
          tunnel: [w734 w737] -> w726
          frame False {
            n286 = Bundle By Name(cluster=w735, "Point File Selected?"=TRUE) -> (w734:T61)
          }
          frame True {
            n287 = Bundle By Name(cluster=w739, "Point File Selected?"=FALSE) -> (w737:T61)
          }
        }
        n288 = call <vilib>:"Add State(s) to Queue__jki_lib_state_machine.vi"("State(s) in (\"\")"=w733) -> ("States Out"=w732:string)  [unwired: 14 in]
      }
      frame "Check Filename Selected" {
        n289 = call <vilib>:"Add State(s) to Queue__jki_lib_state_machine.vi"("State(s) in (\"\")"=w743) -> ("States Out"=w742:string)  [unwired: 14 in]
      }
      frame "Check Exit" {
        n290 = Unbundle By Name(w747) -> ("Test Selected?"=→"Test Selected?":bool, "Point File Selected?"=→"Point File Selected?":bool, "File Name Selected?"=→"File Name Selected?":bool)
        n291 = local read "Control Exit"() -> (w748:bool)
        n292 = case shown="False" w748 {
          tunnel: ["" "Macro: Exit"] -> w749
          frame False {
          }
          frame True {
          }
        }
        n293 = call <vilib>:"Add State(s) to Queue__jki_lib_state_machine.vi"("State(s) in Front (\"\")"=w749, "State(s) in (\"\")"=w752) -> ("States Out"=w751:string)  [unwired: 13 in]
      }
    }
    n294 = local read "Debug?"() -> (w30:bool)
    n295 = case shown="False" w30 {
      tunnel: w33 -> [w46 w49]
      tunnel: w32 -> [_ w48]
      tunnel: [w46 w47] -> w31
      frame False {
      }
      frame True {
        n296 = Build Array (concatenate)(w49, w48) -> (w47:string[])
        "Debug array 2" <- w47
      }
    }
  }
  n297 = while "Plotting SM" {
    shift-right: [w763] -> _
    shift-left: _ -> [w762]
    shift-right: [w766] -> w17
    shift-left: w14 -> [w760]
    shift-right: [w765] -> _
    shift-left: w20 -> [w767]
    shift-right: [w757] -> _
    shift-left: string[] [] -> [w759]
    tunnel: w15 -> [w755]
    stop <- w764 stop-if-true
    # "Plotting SM"
    n298 = call <vilib>:"Parse State Queue__jki_lib_state_machine.vi"("State Queue"=w767, "Error In (no error)"=w760) -> ("Remaining States"=w769:string, "Current State"=w758:string, "Arguments"=w768:string)  [unwired: 11 in]
    n299 = case shown="\"Post Setup Data\"" w758 {
      selector: w758 -> [_ _ w906 _ _ _ _ _ _ _ _ _ _ _ _ _ _ _ _ _ _ _ _ _ _ _ _ _ _ _ _ _ _]
      tunnel: w769 -> [w781 w905 w910 w928 w935 w947 w951 w970 w979 w989 w1005 w1007 w1024 w1052 w1071 w1090 w1106 w1116 w1126 w1140 w1152 w1163 w1189 w1194 w1204 w1208 w1218 w1226 w1311 w1321 w1333 w1369 w1386]
      tunnel: w768 -> [_ _ _ _ _ _ _ _ _ _ _ _ _ _ _ _ _ _ _ _ w1147 w1157 _ _ _ _ _ _ _ _ _ _ _]
      tunnel: w762 -> [w779 w902 w908 w919 w932 w945 w948 _ w975 w986 w1003 w1008 w1014 w1044 w1069 w1088 w1104 w1113 w1122 w1136 w1150 w1159 w1186 w1191 w1201 w1205 w1215 w1224 w1303 w1317 w1326 w1353 w1373]
      tunnel: [w778 w903 w912 w925 errorcluster {"status"=FALSE, "code"=0, "source"=""} ("error out") w944 w949 w967 w973 w987 w994 w1006 w1019 w1045 w1067 w1086 w1097 w1109 w1117 w1137 w1148 w1160 w1187 w1192 w1202 w1206 w1216 w1220 w1304 w1315 w1327 w1367 w1374] -> w766
      tunnel: w760 -> [w777 w903 w911 w925 w930 w944 w949 w967 w976 w987 w999 w1006 w1020 w1046 w1068 w1087 w1103 w1110 w1124 w1138 w1149 w1161 w1187 w1192 w1202 w1206 w1216 w1220 w1306 w1316 w1331 w1367 w1375]
      tunnel: [w780 w904 w909 w927 w934 w946 w950 w969 w978 w988 w1004 w1009 w1023 w1051 w1070 w1089 w1105 w1115 w1125 w1139 w1151 w1162 w1188 w1193 w1203 w1207 w1217 w1225 w1310 w1320 w1332 w1368 w1387] -> w765
      tunnel: [_ _ _ _ _ w943 _ _ _ _ _ _ _ _ _ _ _ _ _ _ _ _ _ _ _ _ _ _ _ _ _ _ _] -> w764
      tunnel: [w776 w902 w908 w926 w932 w945 w948 w968 w975 w986 w991 w1008 w1022 w1044 w1069 w1088 w1104 w1112 w1123 w1136 w1150 w1159 w1186 w1191 w1201 w1205 w1215 w1223 w1309 w1317 w1325 w1348 w1376] -> w763
      tunnel: 1000 ("Timeout") -> [w775 _ _ _ _ _ _ _ _ _ _ _ _ _ _ _ _ _ _ _ _ _ _ _ _ _ _ _ _ _ _ _ _]
      tunnel: w755 -> [w774 _ _ _ _ _ _ _ _ _ _ _ _ _ _ _ _ _ _ _ _ _ _ _ _ _ _ _ _ _ _ _ _]
      frame "", "Event Structure", "Idle" {
        n300 = event shown="[7] <Send Raw Cmd>: User Event" {
          selector: w774 -> [_ _ _ _ _ _ _ _ _ _ _]
          dyn-events: _ -> [_ _ _ _ _ _ _ _ _ _ _]
          timeout: w775 -> [_ _ _ _ _ _ _ _ _ _ _]
          tunnel: w781 -> [w785 w791 w808 w812 w820 w831 w844 w855 w858 w874 w901]
          tunnel: [w784 w790 w808 w812 w819 w832 w845 w856 w859 w873 w900] -> w780
          tunnel: w779 -> [w786 w797 w809 w811 w816 w826 w841 w852 w863 w875 w898]
          tunnel: [w783 w798 w807 w813 w818 w829 w838 w848 w861 w869 w899] -> w778
          tunnel: w777 -> [w783 w798 w807 w813 w818 w829 w834 w848 w861 w870 w899]
          tunnel: [w786 w796 w809 w811 w815 w828 w840 w851 w864 w872 w898] -> w776
          event Timeout {
            n301 = event-data() -> ()  [unwired: 1 in, 1 out]
            n302 = call <vilib>:"Add State(s) to Queue__jki_lib_state_machine.vi"("State(s) in Front (\"\")"="Read Server Data\nUpdate Values\nContactor Settings\nCheck Exit" ("State(s) in Front (\"\")"), "State(s) in (\"\")"=w785) -> ("States Out"=w784:string)  [unwired: 13 in]
          }
          event "Multicolumn Listbox": Value Change; "Multicolumn Listbox": Double Click {
            n303 = event-data() -> ()  [unwired: 1 in, 4 out]
            n304 = Unbundle By Name(w797) -> ("ListBox Selection"=w792:i32[])
            n305 = Index Array(array="Multicolumn Listbox") -> (element=w794:i32)  [unwired: 1 in]
            n306 = Search 1D Array(1D array=w792, element=w794) -> (index of element=w793:i32)  [unwired: 1 in]
            n307 = case shown="0, Default" w793 {
              selector: w793 -> [w799 _]
              tunnel: w794 -> [_ w805]
              tunnel: w792 -> [w802 w804]
              tunnel: [w801 w803] -> w788
              frame 0, Default {
                n308 = Delete From Array(array=w802, length=1, index=w799) -> (array with subset deleted=w801:i32[])  [unwired: 1 out]
              }
              frame -1 {
                n309 = Insert Into Array(array=w804, new element=w805) -> (w803:i32[])  [unwired: 1 in]
              }
            }
            n310 = Sort 1D Array(array=w788) -> (sorted array=w787:i32[])
            n311 = property on="Multicolumn Listbox" class="MCListbox (strict)"("Value"=w788) -> ()  [unwired: 2 in, 2 out]
            n312 = call <vilib>:"Add State(s) to Queue__jki_lib_state_machine.vi"("State(s) in Front (\"\")"="Plot" ("State(s) in Front (\"\")"), "State(s) in (\"\")"=w791) -> ("States Out"=w790:string)  [unwired: 13 in]
            n313 = Bundle By Name(cluster=w797, "ListBox Selection"=w787) -> (w796:T65)
          }
          event "Mixed Signal Graph 2": Mouse Enter {
            n314 = event-data() -> ()  [unwired: 1 in, 4 out]
            n315 = local write "Update Plot"(FALSE ("Update Plot")) -> ()
          }
          event "Mixed Signal Graph 2": Mouse Leave {
            n316 = event-data() -> ()  [unwired: 1 in, 4 out]
            n317 = local write "Update Plot"(TRUE ("Update Plot")) -> ()
          }
          event Value Change {
            n318 = event-data() -> ("NewVal"=w814:T1)  [unwired: 1 in, 5 out]
            n319 = Bundle By Name(cluster=w816, "Tree Selection"=w814) -> (w815:T65)
            n320 = call <vilib>:"Add State(s) to Queue__jki_lib_state_machine.vi"("State(s) in Front (\"\")"="Post Voltage Freq\nPost Ground Leakage\nPost Polarity\nPost Room Setpoints\nCheck Exit\nTree Selection Read" ("State(s) in Front (\"\")"), "State(s) in (\"\")"=w820) -> ("States Out"=w819:string)  [unwired: 13 in]
          }
          event User Event {
            n321 = event-data() -> ()  [unwired: 1 in, 5 out]
            n322 = Unbundle By Name(w826) -> ("Tree Selection"=w825:T1)
            n323 = local read "Point File Path"() -> (w827:path)
            n324 = Path To String(path=w827) -> (string=w824:string)
            n325 = call <vilib>:"Space Constant.vi"() -> ("String"=w822:string)
            n326 = Concatenate Strings(w825, w822, T33 "PF" ("TCP Commands"), w822, w824) -> (w823:string)
            n327 = Bundle By Name(cluster=w826, "Server Write Data"=w823) -> (w828:T65)
            n328 = call <vilib>:"Add State(s) to Queue__jki_lib_state_machine.vi"("State(s) in Front (\"\")"="Write Server Data" ("State(s) in Front (\"\")"), "State(s) in (\"\")"=w831) -> ("States Out"=w832:string)  [unwired: 13 in]
          }
          event User Event {
            n329 = event-data() -> ()  [unwired: 1 in, 5 out]
            n330 = Unbundle By Name(w841) -> ("Tree Selection"=w843:T1, "Station Owner Names"=w837:string[])
            n331 = local read "Data File Path"() -> (w835:path)
            n332 = local read "Setup Info"() -> (w839:string)
            n333 = call "RTS Send File Setup Data.vi"("Error In"=w834, "Setup Info"=w839, "Tree Selection"=w843, "path"=w835) -> ("Error Out"=w833:errorcluster, "File Setup Data"=w842:string)  [unwired: 6 in]
            n334 = call "RTS Get Tech Name.vi"("Error In"=w833, "Station Owner Names Input"=w837, "Setup Info"=w839) -> ("Error Out"=w838:errorcluster, "Station Owner Names Output"=w836:string[])  [unwired: 6 in, 1 out]
            n335 = Bundle By Name(cluster=w841, "Server Write Data"=w842, "Station Owner Names"=w836) -> (w840:T65)
            n336 = call <vilib>:"Add State(s) to Queue__jki_lib_state_machine.vi"("State(s) in Front (\"\")"="Write Server Data" ("State(s) in Front (\"\")"), "State(s) in (\"\")"=w844) -> ("States Out"=w845:string)  [unwired: 13 in]
          }
          event User Event {
            n337 = event-data() -> ()  [unwired: 1 in, 5 out]
            n338 = local read "Raw Command"() -> (w847:string)
            n339 = Unbundle By Name(w852) -> ("Tree Selection"=w854:T1)
            n340 = call <vilib>:"Space Constant.vi"() -> ("String"=w850:string)
            n341 = Concatenate Strings(w854, w850, T33 "CTRL CMD" ("TCP Commands"), w850, w847) -> (w853:string)
            n342 = Bundle By Name(cluster=w852, "Server Write Data"=w853) -> (w851:T65)
            n343 = call <vilib>:"Add State(s) to Queue__jki_lib_state_machine.vi"("State(s) in Front (\"\")"="Write Server Data" ("State(s) in Front (\"\")"), "State(s) in (\"\")"=w855) -> ("States Out"=w856:string)  [unwired: 13 in]
          }
          event User Event {
            n344 = event-data() -> ()  [unwired: 1 in, 5 out]
            n345 = Unbundle By Name(w863) -> ("Tree Selection"=w868:T1)
            n346 = call <vilib>:"Space Constant.vi"() -> ("String"=w866:string)
            n347 = Concatenate Strings(w868, w866, T33 "DOOR CMD" ("TCP Commands"), w866, "Read Door Setup" ("string")) -> (w867:string)
            n348 = Bundle By Name(cluster=w863, "Server Write Data"=w867) -> (w864:T65)
            n349 = call <vilib>:"Add State(s) to Queue__jki_lib_state_machine.vi"("State(s) in Front (\"\")"="Write Server Data" ("State(s) in Front (\"\")"), "State(s) in (\"\")"=w858) -> ("States Out"=w859:string)  [unwired: 13 in]
          }
          event "Save Data": Value Change {
            # "Need to determine which save setting to set. based on chamber selection"
            n350 = event-data() -> ("NewVal"=w871:bool)  [unwired: 1 in, 5 out]
            n351 = case shown="True" w871 {
              tunnel: ["" ("State(s) in Front (\"\")") w882] -> w876
              tunnel: w875 -> [w879 w891]
              tunnel: [w879 w893] -> w872
              tunnel: w870 -> [w877 w886]
              tunnel: [w877 w885] -> w869
              frame False {
              }
              frame True {
                n352 = Unbundle By Name(w891) -> ("Station Owner Names"=w894:string[], "Tree Selection"=w892:T1)
                n353 = local read "Point File Selected?"() -> (w880:bool)
                n354 = local read "Chamber 1 Socket"() -> (w890:string[][])
                n355 = local read "Chamber 2 Socket"() -> (w889:string[][])
                n356 = local read "Chamber 3 Socket"() -> (w888:string[][])
                n357 = local read "Chamber 4 Socket"() -> (w887:string[][])
                n358 = call "RTS Check Save Status.vi"("Chamber 1 Socket"=w890, "Point File Selected?"=w880, "Chamber 2 Socket"=w889, "Chamber 3 Socket"=w888, "Chamber 4 Socket"=w887, "Error In"=w886, "Station Owner Names"=w894, "Tree Selection"=w892) -> ("Next State"=w882:string, "Write Data"=w883:string, "Latest Save State"=→"Latest Save State":bool, "Deselect Log Data"=w881:bool, "Error Out"=w885:errorcluster)  [unwired: 3 in]
                "Deselect Log Data" <- w881
                n359 = case shown="True" w881 {
                  frame False {
                  }
                  frame True {
                    n360 = property on="Save Data" class="Bool (strict)"("Value"=FALSE ("Save Data")) -> ()  [unwired: 2 in, 2 out]
                  }
                }
                n361 = Bundle By Name(cluster=w891, "Server Write Data"=w883) -> (w893:T65)
              }
            }
            n362 = disable-structure shown="Disabled" {
              frame Disabled {
                n363 = local read "File Name Selected?"() -> ()  [unwired: 1 out]
                n364 = local read "Test Selected?"() -> ()  [unwired: 1 out]
              }
              frame Enabled {
              }
            }
            n365 = call <vilib>:"Add State(s) to Queue__jki_lib_state_machine.vi"("State(s) in Front (\"\")"=w876, "State(s) in (\"\")"=w874) -> ("States Out"=w873:string)  [unwired: 13 in]
          }
          event Panel Close? {
            # "Discard the event because we'll close the front panel ourselves in Macro: Exit"
            # "Close Panel button (pressed) Event\n(this executes Macro: Exit to terminate the VI)"
            n366 = event-data() -> ()  [unwired: 1 in, 1 out]
            n367 = call <vilib>:"Add State(s) to Queue__jki_lib_state_machine.vi"("State(s) in Front (\"\")"="Macro: Exit", "State(s) in (\"\")"=w901) -> ("States Out"=w900:string)  [unwired: 13 in]
            n368 = event-data("Discard?"=TRUE) -> ()  [unwired: 1 in, 1 out]
          }
        }
      }
      frame "---------- Core ----------" {
        # "Do not put any code in this frame.\n(it is a separator no-op)"
        n369 = call <vilib>:"Add State(s) to Queue__jki_lib_state_machine.vi"("State(s) in (\"\")"=w905) -> ("States Out"=w904:string)  [unwired: 14 in]
      }
      frame Default {
        w915 = 42 items=["No error", "Argument error", "Memory is full", "Out of zone", "End of file", "File already open", "Generic file I/O error", "File not found", "File permission error", "Disk is full", "Duplicate path", "Too many files open", "System feature not enabled", "Resource file not found", "Cannot add resource", "Resource not found", "Image not found", "Image memory error", "Pen does not exist", "Config type invalid", "Config token not found", "Config parse error", "Config memory error", "Bad external code format", "Bad external code offset", "External code not present", "Null window", "Destroy window error", "Null menu", "Print aborted", "Bad print record", "Print driver error", "Windows error during printing", "Memory error during printing", "Print dialog error", "Generic print error", "Invalid device refnum", "Device not found", "Device parameter error", "Device unit error", "Cannot open device", "Device call aborted", "Generic error", "Cancelled by user", "Object ID too low", "Object ID too high", "Object not in heap", "Unknown heap", "Unknown object (invalid DefProc)", "Unknown object (DefProc not in table)", "Message out of range", "Invalid (null) method", "Unknown message", "Manager call not supported", "Bad address", "Network operation in progress", "Network operation timed out", "Connection is busy", "Network attribute not supported", "Network error", "Address in use", "System out of memory", "Connection aborted", "Connection refused", "Not connected", "Already connected", "Connection closed", "Initialization error (interapplication manager)", "Bad occurrence", "Wait on unbound occurrence handler", "Occurrence queue overflow", "Datalog type conflict", "Unused", "Unrecognized type (interapplication manager)", "Memory corrupt", "Failed to make temporary DLL", "Old CIN version", "Drag socket not found", "Failed to load drop-object", "Failed to register OLE object", "Failed to release OLE object", "Format specifier type mismatch", "Unknown format specifier", "Too few format specifiers", "Too many format specifiers", "Scan failed", "Newer CIN version", "Error converting to variant", "Runtime menu error", "Password tampered", "Variant attribute not found", "Incompatible variant data type", "Event data is not available", "Event Store is not present", "Occurrence is not found", "Event Queue is not created", "Event info is not available", "Refnum passed is NULL", "Error retrieving Class GUID", "Error retrieving CoClass GUID", "Error retrieving TypeLib GUID.", "Bad built application magic bytes.", "Specific driver is different from the specific driver associated with the Logical Name.", "There is no session opened to the class driver.", "Max Error", "MAX - Error with config objects", "MAX - Error loading configuration", "MAX - Group not supported"]
        # "Current State"
        # "Do not delete, rename, or modify this frame.\n(this is used to capture unhandled states and typos)"
        # "Handle mistyped state name (developer tool)"
        n370 = Format Into String(format string="Software Exception: Unhandled State \"%s\"." ("message"), error in=w911, w906) -> (resulting string=w914:string, error out=w913:errorcluster)  [unwired: 1 in]
        n371 = call <vilib>:"Error Cluster From Error Code.vi"("show call chain? (False)"=TRUE, "error in (no error)"=w913, "error message (\"\")"=w914, "error code (0)"=w915) -> ("error out"=w912:errorcluster)  [unwired: 5 in]
        n372 = call <vilib>:"Add State(s) to Queue__jki_lib_state_machine.vi"("State(s) in (\"\")"=w910) -> ("States Out"=w909:string)  [unwired: 14 in]
      }
      frame "Initialize Core Data" {
        # "originally closed?"
        # "exe?"
        # "If panel starts closed or is an EXE, then close it when we exit"
        n373 = property class="VI"() -> ("Front Panel.Open"=w924:bool)  [unwired: 2 in, 2 out]
        n374 = property class="App"() -> ("App.Kind"=w923:T37)  [unwired: 2 in, 2 out]
        n375 = Not(x=w924) -> (.not. x?=w921:bool)
        n376 = Equal?(x=w923, y=T37."Run Time System" ("Application:Kind")) -> (x = y?=w920:bool)
        n377 = Or(x=w921, y=w920) -> (x .or. y?=w918:bool)
        n378 = control-ref of="Current VI Reference"() -> (w917:refnum<vi>)
        n379 = Bundle By Name(cluster=w919, "Core.Current VI Reference"=w917, "Core.Close Panel on Exit?"=w918) -> (w926:T65)
        n380 = call <vilib>:"Add State(s) to Queue__jki_lib_state_machine.vi"("State(s) in (\"\")"=w928) -> ("States Out"=w927:string)  [unwired: 14 in]
      }
      frame "Error Handler" {
        # "Certain error codes can occur if the server VI closes the connection. In these cases, ignore the potential errors that can occur, and instead pop up a dialog indicating that the server closed the connection."
        # "Unhandled Error -- Display it"
        # "Handle any errors here.\nYou can also output any states to clean-up after errors occur"
        # "Clear error"
        n381 = case shown="Error" w930 {
          selector: w930 -> [w936 w938]
          tunnel: [w936 w937] -> w929
          frame No Error {
          }
          frame Error {
            n382 = Unbundle By Name(w938) -> ("code"=w939:i32)
            n383 = case shown="Default" w939 {
              tunnel: w938 -> [w940 _]
              tunnel: [w940 w942] -> w937
              frame Default {
              }
              frame 62, 64, 66 {
                w942 = errorcluster {"status"=FALSE, "code"=0, "source"=""}  # No error
                n384 = One Button Dialog(message="Server Closed") -> ()  [unwired: 1 in, 1 out]
              }
            }
          }
        }
        n385 = call <vilib>:"General Error Handler.vi"("error in (no error)"=w929) -> ()  [unwired: 10 in, 5 out]
        n386 = call <vilib>:"Add State(s) to Queue__jki_lib_state_machine.vi"("State(s) in Front (\"\")"="/* Post Error States", "State(s) in (\"\")"=w935) -> ("States Out"=w934:string)  [unwired: 13 in]
      }
      frame "Exit" {
        w943 = TRUE
        # "Do not put any code in this frame.\n(No errors that occur here will be handled.)"
        n387 = call <vilib>:"Add State(s) to Queue__jki_lib_state_machine.vi"("State(s) in (\"\")"=w947) -> ("States Out"=w946:string)  [unwired: 14 in]
        "Control Exit" <- w943
      }
      frame "---------- Data ----------" {
        # "Do not put any code in this frame.\n(It is a separator no-op. You can make a copy of this frame to create a new Data frame)"
        n388 = call <vilib>:"Add State(s) to Queue__jki_lib_state_machine.vi"("State(s) in (\"\")"=w951) -> ("States Out"=w950:string)  [unwired: 14 in]
      }
      frame "Data: Initialize" {
        w954 = string[] []  # Custom Titles
        w955 = string[] []  # Listbox Item Names
        w956 = string[][] []  # Chamber Data
        w957 = string[] ["", "", "", "", "", "", "", "", "", "", "", "", "", "", "", "", "", "", "", "", "", "", "", "", "", "", "", "", "", "", "", ""]  # Station Owner Names
        w960 = ""  # Server Write Data
        w963 = string[] []  # Full Item Names
        w964 = dbl[][] []  # All Data
        w965 = i32[] []  # ListBox Selection
        w966 = T62 {"Current VI Reference"=refnum, "Close Panel on Exit?"=FALSE}  # Core
        # "Initialize the shift-register data, here.\n(data names are defined by what you wire into the bundle function)"
        n389 = property on="Multicolumn Listbox" class="MCListbox (strict)"("Value"=w965) -> ()  [unwired: 2 in, 2 out]
        n390 = local write "Tab Control"(T16."Trending Data" ("Tab Control")) -> ()
        n391 = call <vilib>:"Add State(s) to Queue__jki_lib_state_machine.vi"("State(s) in (\"\")"=w970) -> ("States Out"=w969:string)  [unwired: 14 in]
        n392 = Bundle("Core"=w966, "ListBox Selection"=w965, "All Data"=w964, "Full Item Names"=w963, "CSV Data Save"="CSV Data Save", "Data"=T63 {"Clients"=[], "Listener"=refnum, "Data Array"=[]}, "Tree Selection"="Tree Selection", "RTS Config Setup"=T6 {"Wago RTS"={"Disable"=0, "Interval"=0, "Controller"=0, "Address"=0, "IP Address"="", "AtoDmax"=0, "FullScale"=0, "VoltageType"=0, "Window1"=0, "Control1"=0, "Window2"=0, "Control2"=0}, "APLUS Array"=[], "Yokogawa MX100 RTS Array"=[], "Replay Server"=[], "Server Configuration Array"=[], "Station Settings"={"Point Files"={"Point File 1"=path "", "Point File 2"=path "", "Point File 3"=path "", "Point File 4"=path "", "Point File 5"=path "", "Point File 6"=path "", "Point File 7"=path "", "Point File 8"=path ""}, "Save Status"={"Save Status 1"=FALSE, "Save Status 2"=FALSE, "Save Status 3"=FALSE, "Save Status 4"=FALSE, "Save Status 5"=FALSE, "Save Status 6"=FALSE, "Save Status 7"=FALSE, "Save Status 8"=FALSE}, "Setup Info"={"Setup Info Station 1"=[], "Setup Info Station 2"=[], "Setup Info Station 3"=[], "Setup Info Station 4"=[], "Setup Info Station 5"=[], "Setup Info Station 6"=[], "Setup Info Station 7"=[], "Setup Info Station 8"=[]}, "Chamber Test Pattern"={" Pattern 1"=path "", "Pattern 2"=path "", "Pattern 3"=path "", "Pattern 4"=path "", "Pattern 5"=path "", "Pattern 6"=path "", "Pattern 7"=path "", "Pattern 8"=path ""}}}, "Server Write Data"=w960, "Station Owner Names"=w957, "Chamber Data"=w956, "Listbox Item Names"=w955, "Custom Titles"=w954, "Filepath"="Filepath") -> (w968:T65)  [unwired: 1 in]
      }
      frame "Data: Cleanup" {
        # "Cleanup any data and references, here.\n(this is called automatically, by the Macro: Exit)"
        n393 = Unbundle By Name(w975) -> ("Data.Clients"=w972:refnum<k5>[], "Core.Current VI Reference"=w977:refnum<vi>)
        n394 = Close Reference(reference=w977, error in (no error)=w976) -> (error out=w971:errorcluster)
        n395 = call <vilib>:"Simple Error Handler.vi"("error in (no error)"=w971) -> ("error out"=w974:errorcluster)  [unwired: 1 in, 7 out]
        n396 = for {
          tunnel: w972 -> [w981] mode=indexing
          shift-right: [w982] -> w973
          shift-left: w974 -> [w983]
          n397 = TCP Write(connection ID=w981, data in="Q", error in (no error)=w983) -> (connection ID out=w985:refnum<k5>, error out=w984:errorcluster)  [unwired: 2 out]
          n398 = TCP Close Connection(connection ID=w985, error in (no error)=w984) -> (error out=w982:errorcluster)  [unwired: 2 out]
        }
        n399 = call <vilib>:"Add State(s) to Queue__jki_lib_state_machine.vi"("State(s) in (\"\")"=w979) -> ("States Out"=w978:string)  [unwired: 14 in]
      }
      frame "---------- UI ----------" {
        n400 = call <vilib>:"Add State(s) to Queue__jki_lib_state_machine.vi"("State(s) in (\"\")"=w989) -> ("States Out"=w988:string)  [unwired: 14 in]
      }
      frame "UI: Initialize" {
        n401 = Current VI's Path() -> (path=w1002:path)
        n402 = call "UTILITY This VIs Path.vi"("path"=w1002, "error in (no error)"=w999) -> ("Folder Path"=w998:path, "FileVersionInfo Out"=w1001:T54, "error out"=w995:errorcluster)  [unwired: 7 in, 4 out]
        "Base Path" <- w998
        n403 = Unbundle By Name(w1001) -> ("FileVersion"=→"File  Version":string)
        n404 = Bundle By Name(cluster=w1003, "Filepath.General Setup Paths.Tool Base Path"=w998) -> (w992:T65)
        n405 = Unbundle By Name(w992) -> ("Filepath"=w993:T2)
        n406 = call "Save File DOE File Setup.vi"("Filepath In"=w993, "error in (no error)"=w995, "Config State"=Save_File_DOE_Configuration_State."Load Config", "LV Program"=Save_File_DOE_LabView_Program."Refrigeration") -> ("Filepath Out"=w990:T2, "error out"=w994:errorcluster)  [unwired: 13 in, 1 out]
        n407 = Bundle By Name(cluster=w992, "Filepath"=w990) -> (w991:T65)
        n408 = local write "Filepath"(w990) -> ()
        n409 = call <vilib>:"Add State(s) to Queue__jki_lib_state_machine.vi"("State(s) in (\"\")"=w1005) -> ("States Out"=w1004:string)  [unwired: 14 in]
      }
      frame "Load Config File" {
        n410 = call <vilib>:"Add State(s) to Queue__jki_lib_state_machine.vi"("State(s) in (\"\")"=w1007) -> ("States Out"=w1009:string)  [unwired: 14 in]
      }
      frame "Read Config Files" {
        # "The data file path is referenced \nfrom the server..kinda confusing\nbut it a client server app"
        # "When i ramp up all chambers.\n\nthis will probably need to be an\narray to accomodate each chamber\nconfig file (corresponds with multiple\nTCP ports open)"
        n411 = Unbundle By Name(w1014) -> ("Filepath.General Setup Paths.Data Folder Path"=w1017:path)
        n412 = Strip Path(path=w1017) -> (stripped path=w1016:path)  [unwired: 1 out]
        n413 = Build Path(base path=w1016, name or relative path="Haier RTS") -> (appended path=w1013:path)
        n414 = Bundle By Name(cluster=w1014, "Filepath.General Setup Paths.General Startup Config Path"=w1013) -> (w1012:T65)
        n415 = Unbundle By Name(w1012) -> ("Filepath"=w1010:T2, "Filepath.General Setup Paths.General Startup Config Path"=w1011:path)
        n416 = local write "Filepath"(w1010) -> ()
        n417 = call "RTS Read Configuration Files.vi"("System Number"=T64 "Sys1", "Error In"=w1020, "Core System Path"=w1011) -> ("Error Out"=w1019:errorcluster, "RTS Config Setup Output"=w1018:T6)  [unwired: 7 in]
        "RTS Config Setup Output" <- w1018
        n418 = call <vilib>:"Add State(s) to Queue__jki_lib_state_machine.vi"("State(s) in (\"\")"=w1024) -> ("States Out"=w1023:string)  [unwired: 14 in]
        n419 = Bundle By Name(cluster=w1012, "RTS Config Setup"=w1018) -> (w1022:T65)
      }
      frame "Post Voltage Freq" {
        w1025 = RTS_Reset_Watt_Hours."" ("Wh Reset 1")
        n420 = local read "Chamber 1 Socket"() -> (w1050:string[][])
        n421 = local read "Chamber 2 Socket"() -> (w1049:string[][])
        n422 = local read "Chamber 3 Socket"() -> (w1048:string[][])
        n423 = local read "Chamber 4 Socket"() -> (w1047:string[][])
        n424 = Unbundle By Name(w1044) -> ("Tree Selection"=w1043:T1)
        n425 = property on="Wh Reset 1" class="Enum (strict)"("Value"=w1025) -> ()  [unwired: 2 in, 2 out]
        n426 = property on="Wh Reset 2" class="Enum (strict)"("Value"=w1025) -> ()  [unwired: 2 in, 2 out]
        n427 = property on="Wh Reset 3" class="Enum (strict)"("Value"=w1025) -> ()  [unwired: 2 in, 2 out]
        n428 = property on="Wh Reset 4" class="Enum (strict)"("Value"=w1025) -> ()  [unwired: 2 in, 2 out]
        n429 = property on="Wh Reset 5" class="Enum (strict)"("Value"=w1025) -> ()  [unwired: 2 in, 2 out]
        n430 = property on="Wh Reset 6" class="Enum (strict)"("Value"=w1025) -> ()  [unwired: 2 in, 2 out]
        n431 = property on="Wh Reset 7" class="Enum (strict)"("Value"=w1025) -> ()  [unwired: 2 in, 2 out]
        n432 = property on="Wh Reset 8" class="Enum (strict)"("Value"=w1025) -> ()  [unwired: 2 in, 2 out]
        n433 = call "RTS Post Voltage Frequency.vi"("Chamber 1 Socket"=w1050, "Chamber 2 Socket"=w1049, "Chamber 3 Socket"=w1048, "Chamber 4 Socket"=w1047, "Error In"=w1046, "Tree Selection"=w1043) -> ("Voltage & Freq"=w1042:T66, "Error Out"=w1045:errorcluster)  [unwired: 12 in]
        n434 = Unbundle By Name(w1042) -> ("Voltage 1"=w1041:dbl, "Voltage 2"=w1040:dbl, "Voltage 3"=w1039:dbl, "Voltage 4"=w1038:dbl, "Voltage 5"=w1037:dbl, "Voltage 6"=w1036:dbl, "Voltage 7"=w1035:dbl, "Voltage 8"=w1034:dbl, "Frequency 1"=w1033:T19, "Frequency 2"=w1032:T19, "Frequency 3"=w1031:T19, "Frequency 4"=w1030:T19, "Frequency 5"=w1029:T19, "Frequency 6"=w1028:T19, "Frequency 7"=w1027:T19, "Frequency 8"=w1026:T19)
        n435 = local write "Voltage"(w1041) -> ()
        n436 = local write "Voltage 2"(w1040) -> ()
        n437 = local write "Voltage 3"(w1039) -> ()
        n438 = local write "Voltage 4"(w1038) -> ()
        n439 = local write "Voltage 5"(w1037) -> ()
        n440 = local write "Voltage 6"(w1036) -> ()
        n441 = local write "Voltage 7"(w1035) -> ()
        n442 = local write "Voltage 8"(w1034) -> ()
        n443 = local write "Frequency"(w1033) -> ()
        n444 = local write "Frequency 2"(w1032) -> ()
        n445 = local write "Frequency 3"(w1031) -> ()
        n446 = local write "Frequency 4"(w1030) -> ()
        n447 = local write "Frequency 5"(w1029) -> ()
        n448 = local write "Frequency 6"(w1028) -> ()
        n449 = local write "Frequency 7"(w1027) -> ()
        n450 = local write "Frequency 8"(w1026) -> ()
        n451 = call <vilib>:"Add State(s) to Queue__jki_lib_state_machine.vi"("State(s) in (\"\")"=w1052) -> ("States Out"=w1051:string)  [unwired: 14 in]
      }
      frame "Post Ground Leakage" {
        # "Measure Ground Leakage Current = 78"
        n452 = local read "Chamber 1 Socket"() -> (w1064:string[][])
        n453 = local read "Chamber 2 Socket"() -> (w1063:string[][])
        n454 = local read "Chamber 3 Socket"() -> (w1062:string[][])
        n455 = local read "Chamber 4 Socket"() -> (w1061:string[][])
        n456 = Unbundle By Name(w1069) -> ("Tree Selection"=w1065:T1)
        n457 = call "RTS Relay Status.vi"("Chamber 1 Socket"=w1064, "Tree Selection"=w1065, "Chamber 2 Socket"=w1063, "Chamber 3 Socket"=w1062, "Chamber 4 Socket"=w1061, "error in (no error)"=w1068, "Extract Column"=78) -> ("Station 1"=w1060:i32, "Station 2"=w1059:i32, "Station 3"=w1058:i32, "Station 4"=w1057:i32, "Station 5"=w1056:i32, "Station 6"=w1055:i32, "Station 8"=w1053:i32, "Station 7"=w1054:i32, "error out"=w1067:errorcluster)
        n458 = property on="Ground Leakage 1" class="Enum (strict)"("Value"=w1060) -> ()  [unwired: 2 in, 2 out]
        n459 = property on="Ground Leakage 2" class="Enum (strict)"("Value"=w1059) -> ()  [unwired: 2 in, 2 out]
        n460 = property on="Ground Leakage 3" class="Enum (strict)"("Value"=w1058) -> ()  [unwired: 2 in, 2 out]
        n461 = property on="Ground Leakage 4" class="Enum (strict)"("Value"=w1057) -> ()  [unwired: 2 in, 2 out]
        n462 = property on="Ground Leakage 5" class="Enum (strict)"("Value"=w1056) -> ()  [unwired: 2 in, 2 out]
        n463 = property on="Ground Leakage 6" class="Enum (strict)"("Value"=w1055) -> ()  [unwired: 2 in, 2 out]
        n464 = property on="Ground Leakage 7" class="Enum (strict)"("Value"=w1054) -> ()  [unwired: 2 in, 2 out]
        n465 = property on="Ground Leakage 8" class="Enum (strict)"("Value"=w1053) -> ()  [unwired: 2 in, 2 out]
        n466 = call <vilib>:"Add State(s) to Queue__jki_lib_state_machine.vi"("State(s) in (\"\")"=w1071) -> ("States Out"=w1070:string)  [unwired: 14 in]
      }
      frame "Post Polarity" {
        # "Ground Line-76"
        n467 = local read "Chamber 1 Socket"() -> (w1085:string[][])
        n468 = local read "Chamber 2 Socket"() -> (w1084:string[][])
        n469 = local read "Chamber 3 Socket"() -> (w1083:string[][])
        n470 = local read "Chamber 4 Socket"() -> (w1082:string[][])
        n471 = Unbundle By Name(w1088) -> ("Tree Selection"=w1081:T1)
        n472 = call "RTS Relay Status.vi"("Chamber 1 Socket"=w1085, "Tree Selection"=w1081, "Chamber 2 Socket"=w1084, "Chamber 3 Socket"=w1083, "Chamber 4 Socket"=w1082, "error in (no error)"=w1087, "Extract Column"=76) -> ("Station 1"=w1079:i32, "Station 2"=w1078:i32, "Station 3"=w1077:i32, "Station 4"=w1076:i32, "Station 5"=w1075:i32, "Station 6"=w1074:i32, "Station 8"=w1072:i32, "Station 7"=w1073:i32, "error out"=w1086:errorcluster)
        n473 = property on="Station 1 - Polarity" class="Enum (strict)"("Value"=w1079) -> ()  [unwired: 2 in, 2 out]
        n474 = property on="Station 2 - Polarity" class="Enum (strict)"("Value"=w1078) -> ()  [unwired: 2 in, 2 out]
        n475 = property on="Station 3 - Polarity" class="Enum (strict)"("Value"=w1077) -> ()  [unwired: 2 in, 2 out]
        n476 = property on="Station 4 - Polarity" class="Enum (strict)"("Value"=w1076) -> ()  [unwired: 2 in, 2 out]
        n477 = property on="Station 5 - Polarity" class="Enum (strict)"("Value"=w1075) -> ()  [unwired: 2 in, 2 out]
        n478 = property on="Station 6 - Polarity" class="Enum (strict)"("Value"=w1074) -> ()  [unwired: 2 in, 2 out]
        n479 = property on="Station 7 - Polarity" class="Enum (strict)"("Value"=w1073) -> ()  [unwired: 2 in, 2 out]
        n480 = property on="Station 8 - Polarity" class="Enum (strict)"("Value"=w1072) -> ()  [unwired: 2 in, 2 out]
        n481 = call <vilib>:"Add State(s) to Queue__jki_lib_state_machine.vi"("State(s) in (\"\")"=w1090) -> ("States Out"=w1089:string)  [unwired: 14 in]
      }
      frame "Post Room Setpoints" {
        # "Room Setpoint Temperature-45\nRoom Setpoint Humidity-46\nRoom Setpoint Cool Temperature-50\nRoom Setpoint Dehumidification Temperature-51"
        n482 = Unbundle By Name(w1104) -> ("Tree Selection"=w1091:T1)
        n483 = local read "Chamber 1 Socket"() -> (w1096:string[][])
        n484 = local read "Chamber 2 Socket"() -> (w1095:string[][])
        n485 = local read "Chamber 3 Socket"() -> (w1094:string[][])
        n486 = local read "Chamber 4 Socket"() -> (w1093:string[][])
        n487 = call "RTS Extract Room Setpoint Status.vi"("Chamber 1 Socket"=w1096, "Tree Selection in"=w1091, "Chamber 2 Socket"=w1095, "Chamber 3 Socket"=w1094, "Chamber 4 Socket"=w1093, "error in (no error)"=w1103) -> ("Room Setpoint Temperature"=w1102:dbl, "Room Setpoint Humidity"=w1101:dbl, "Room Setpoint Cool Temperature"=w1100:dbl, "Room Setpoint Dehumidification Temperature"=w1099:dbl, "error out"=w1098:errorcluster)  [unwired: 5 in]
        n488 = property on="Room Setpoint Temperature (*RM Dry Set P1)" class="DigNum (strict)"("Value"=w1102) -> ()  [unwired: 2 in, 2 out]
        n489 = property on="Room Setpoint Humidity (*RM Hum Set P1)" class="DigNum (strict)"("Value"=w1101) -> ()  [unwired: 2 in, 2 out]
        n490 = property on="Room Cool Temperature (*RM Cool Setp 1)" class="DigNum (strict)"("Value"=w1100) -> ()  [unwired: 2 in, 2 out]
        n491 = property on="Room Dehum Temperature (*RM De Hum Set P1)" class="DigNum (strict)"("Value"=w1099) -> ()  [unwired: 2 in, 2 out]
        n492 = call "RTS Find Save State.vi"("Chamber 1 Socket in"=w1096, "Chamber 2 Socket in"=w1095, "Chamber 3 Socket in"=w1094, "Chamber 4 Socket in"=w1093, "Error In"=w1098, "Tree Selection in"=w1091) -> ("Current Save State"=w1092:string, "Error Out"=w1097:errorcluster)  [unwired: 3 in, 5 out]
        n493 = case shown="\"TRUE\"" w1092 {
          frame "FALSE", Default {
            n494 = property on="Save Data" class="Bool (strict)"("Value"=FALSE ("Save Data")) -> ()  [unwired: 2 in, 2 out]
          }
          frame "TRUE" {
            n495 = property on="Save Data" class="Bool (strict)"("Value"=TRUE ("Save Data")) -> ()  [unwired: 2 in, 2 out]
          }
        }
        n496 = call <vilib>:"Add State(s) to Queue__jki_lib_state_machine.vi"("State(s) in (\"\")"=w1106) -> ("States Out"=w1105:string)  [unwired: 14 in]
      }
      frame "Post Setup Data" {
        n497 = Unbundle By Name(w1113) -> ("RTS Config Setup.Station Settings"=w1114:T12)
        n498 = call "RTS Post Client Setup Data.vi"("Error In"=w1110, "Station Settings In"=w1114) -> ("Error Out"=w1109:errorcluster, "Station Settings Out"=w1111:T12)  [unwired: 8 in]
        n499 = Bundle By Name(cluster=w1113, "RTS Config Setup.Station Settings"=w1111) -> (w1112:T65)
        n500 = call <vilib>:"Add State(s) to Queue__jki_lib_state_machine.vi"("State(s) in (\"\")"=w1116) -> ("States Out"=w1115:string)  [unwired: 14 in]
      }
      frame "Open TCP Port" {
        # "Need to delete\nwhen i run\nall chambers\nat same time"
        n501 = Unbundle By Name(w1122) -> ("RTS Config Setup.Server Configuration Array"=w1121:T11[])
        n502 = for {
          N: 1 -> [_]
          tunnel: [w1132] -> w1120 mode=indexing
          shift-right: [w1133] -> w1118
          shift-left: w1124 -> [w1134]
          tunnel: w1121 -> [w1130] mode=indexing
          (unwired) "localhost"  # address
          w1129 = "10.83.202.5"  # address
          # "Will need to get IP address\nof remote server"
          n503 = Unbundle By Name(w1130) -> ("TcpIP"=w1131:u16)
          n504 = TCP Open Connection(address=w1129, remote port or service name=w1131, error in (no error)=w1134) -> (connection ID=w1132:refnum<k5>, error out=w1133:errorcluster)  [unwired: 2 out]
        }
        n505 = Bundle By Name(cluster=w1122, "Data.Clients"=w1120) -> (w1123:T65)
        n506 = flat-sequence {
          tunnel: w1118 -> [w1127]
          tunnel: [w1127] -> w1117
          frame #0 {
            "Start UI Loop" <- TRUE ("Start UI Loop")
          }
        }
        n507 = call <vilib>:"Add State(s) to Queue__jki_lib_state_machine.vi"("State(s) in (\"\")"=w1126) -> ("States Out"=w1125:string)  [unwired: 14 in]
      }
      frame "Close TCP Port" {
        n508 = Unbundle By Name(w1136) -> ("Data.Clients"=w1135:refnum<k5>[])
        n509 = for {
          tunnel: w1135 -> [w1141] mode=indexing
          shift-right: [w1142] -> w1137
          shift-left: w1138 -> [w1143]
          n510 = TCP Write(connection ID=w1141, data in="Q", error in (no error)=w1143) -> (connection ID out=w1146:refnum<k5>, error out=w1145:errorcluster)  [unwired: 2 out]
          n511 = TCP Close Connection(connection ID=w1146, error in (no error)=w1145) -> (error out=w1142:errorcluster)  [unwired: 2 out]
        }
        n512 = call <vilib>:"Add State(s) to Queue__jki_lib_state_machine.vi"("State(s) in (\"\")"=w1140) -> ("States Out"=w1139:string)  [unwired: 14 in]
      }
      frame "UI: Cursor Set" {
        # "Argument"
        n513 = case shown="\"Idle\", Default" w1147 {
          tunnel: w1149 -> [w1154 w1156]
          tunnel: [w1153 w1155] -> w1148
          frame "Idle", Default {
            n514 = call <vilib>:"Unset Busy.vi"("error in (no error)"=w1154) -> ("error out"=w1153:errorcluster)  [unwired: 10 in]
          }
          frame "Busy" {
            n515 = call <vilib>:"Set Busy.vi"("error in (no error)"=w1156) -> ("error out"=w1155:errorcluster)  [unwired: 9 in, 1 out]
          }
        }
        n516 = call <vilib>:"Add State(s) to Queue__jki_lib_state_machine.vi"("State(s) in (\"\")"=w1152) -> ("States Out"=w1151:string)  [unwired: 14 in]
      }
      frame "UI: Front Panel State" {
        # "Argument"
        n517 = Unbundle By Name(w1159) -> ("Core.Current VI Reference"=w1158:refnum<vi>)
        n518 = case shown="\"Open\", Default" w1157 {
          tunnel: w1161 -> [w1167 w1180]
          tunnel: [w1169 w1181] -> w1160
          tunnel: w1158 -> [w1168 w1178]
          frame "Open", Default {
            n519 = property class="VI"(reference=w1168, error in=w1167) -> (reference out=w1165:refnum<vi>, error out=w1166:errorcluster, "Front Panel.Open"=w1164:bool)
            n520 = case shown="True" w1164 {
              tunnel: [w1172 w1175] -> w1169
              tunnel: w1166 -> [w1171 w1175]
              tunnel: w1165 -> [w1170 _]
              frame False {
                n521 = invoke class="VI" method="FP.Open"(reference=w1170, error in=w1171, "Activate"=TRUE, "State"=T38."Standard") -> (error out=w1172:errorcluster)  [unwired: 1 in, 4 out]
              }
              frame True {
              }
            }
          }
          frame "Close" {
            n522 = property class="VI"(reference=w1178, error in=w1180) -> (reference out=w1177:refnum<vi>, error out=w1179:errorcluster, "Front Panel.Open"=w1176:bool)
            n523 = case shown="True" w1176 {
              tunnel: [w1182 w1185] -> w1181
              tunnel: w1179 -> [w1182 w1184]
              tunnel: w1177 -> [_ w1183]
              frame False {
              }
              frame True {
                n524 = invoke class="VI" method="FP.Close"(reference=w1183, error in=w1184) -> (error out=w1185:errorcluster)  [unwired: 1 in, 2 out]
              }
            }
          }
        }
        n525 = call <vilib>:"Add State(s) to Queue__jki_lib_state_machine.vi"("State(s) in (\"\")"=w1163) -> ("States Out"=w1162:string)  [unwired: 14 in]
      }
      frame "---------- Macro ----------" {
        n526 = call <vilib>:"Add State(s) to Queue__jki_lib_state_machine.vi"("State(s) in (\"\")"=w1189) -> ("States Out"=w1188:string)  [unwired: 14 in]
      }
      frame "Macro: Initialize" {
        w1190 = "Data: Initialize\nInitialize Core Data\nUI: Initialize\nUI: Front Panel State >> Open\nRead Config Files\nOpen TCP Port"  # Data: Initialize Initialize Core Data UI: Initialize UI: Front Panel State >> Open Read Config Files Open TCP Port
        n527 = call <vilib>:"Add State(s) to Queue__jki_lib_state_machine.vi"("State(s) in Front (\"\")"=w1190, "State(s) in (\"\")"=w1194) -> ("States Out"=w1193:string)  [unwired: 13 in]
      }
      frame "Macro: Exit" {
        n528 = Unbundle By Name(w1201) -> ("Core.Close Panel on Exit?"=w1200:bool)
        n529 = Select(t="UI: Front Panel State >> Close", s=w1200, f="") -> (s? t:f=w1197:string)
        n530 = call <vilib>:"Add State(s) to Queue__jki_lib_state_machine.vi"("State(s) in (\"\")"=w1197, "State(s) at Back (\"\")"="Data: Cleanup\nExit") -> ("States Out"=w1195:string)  [unwired: 13 in]
        n531 = call <vilib>:"Add State(s) to Queue__jki_lib_state_machine.vi"("State(s) in Front (\"\")"=w1195, "State(s) in (\"\")"=w1204) -> ("States Out"=w1203:string)  [unwired: 13 in]
      }
      frame "---------- New Category ----------" {
        n532 = call <vilib>:"Add State(s) to Queue__jki_lib_state_machine.vi"("State(s) in (\"\")"=w1208) -> ("States Out"=w1207:string)  [unwired: 14 in]
      }
      frame "Plot" {
        n533 = Unbundle By Name(w1215) -> ("All Data"=w1211:dbl[][], "ListBox Selection"=w1214:i32[], "Full Item Names"=w1212:string[], "Listbox Item Names"=w1210:string[], "Custom Titles"=w1209:string[])
        n534 = call "Plotting Assemble.vi"("Custom Titles"=w1209, "Listbox Item Names"=w1210, "Full Item Names"=w1212, "OldVal"=w1214, "All Data"=w1211) -> ("Mixed Signal Graph"=→"Mixed Signal Graph 2":T17)  [unwired: 5 in, 1 out]
        n535 = call <vilib>:"Add State(s) to Queue__jki_lib_state_machine.vi"("State(s) in (\"\")"=w1218) -> ("States Out"=w1217:string)  [unwired: 14 in]
      }
      frame "Read Server Data" {
        n536 = Unbundle By Name(w1224) -> ("Data.Clients"=w1222:refnum<k5>[])
        n537 = for {
          tunnel: w1222 -> [w1229] mode=indexing
          tunnel: [w1228] -> w1221 mode=indexing
          i -> [w1227]
          n538 = Equal?(x=w1229, y=refnum<k5> refnum ("x")) -> (x = y?=w1230:bool)
          n539 = case shown="False" w1230 {
            tunnel: [w1233 w1287] -> w1228
            tunnel: w1229 -> [w1234 w1287]
            tunnel: w1227 -> [w1232 _]
            frame False {
              n540 = case shown="0, Default" w1232 {
                tunnel: w1234 -> [w1239 w1253 w1265 w1278]
                tunnel: [w1238 w1252 w1264 w1277] -> w1233
                frame 0, Default {
                  n541 = call "RTS Read TCP Command.vi"("Client Side?"=TRUE, "TCP Network Connection in"=w1239) -> ("TCP Command"=w1240:string, "TCP Network Connection out"=w1238:refnum<k5>, "Custom CMD?"=w1236:bool)  [unwired: 6 in, 1 out]
                  n542 = case shown="False" w1236 {
                    tunnel: w1240 -> [w1243 _]
                    tunnel: ["" ("Custom CMD State") "Post Setup Data" ("Custom CMD State")] -> w1235
                    frame False {
                      n543 = Spreadsheet String To Array(delimiter (Tab)=",", format string="%s", spreadsheet string=w1243, array type (2D Dbl)=string[][] []) -> (array=→"Chamber 1 Socket":string[][])
                    }
                    frame True {
                    }
                  }
                  n544 = local write "Custom CMD State"(w1235) -> ()
                }
                frame 1 {
                  n545 = call "RTS Read TCP Command.vi"("Client Side?"=TRUE, "TCP Network Connection in"=w1253) -> ("TCP Command"=w1251:string, "TCP Network Connection out"=w1252:refnum<k5>, "Custom CMD?"=w1249:bool)  [unwired: 6 in, 1 out]
                  n546 = case shown="False" w1249 {
                    tunnel: w1251 -> [w1256 _]
                    tunnel: ["" ("Custom CMD State") "Post Setup Data" ("Custom CMD State")] -> w1248
                    frame False {
                      n547 = Spreadsheet String To Array(delimiter (Tab)=",", format string="%s", spreadsheet string=w1256, array type (2D Dbl)=string[][] []) -> (array=→"Chamber 2 Socket":string[][])
                    }
                    frame True {
                    }
                  }
                  n548 = local write "Custom CMD State"(w1248) -> ()
                }
                frame 2 {
                  n549 = call "RTS Read TCP Command.vi"("Client Side?"=TRUE, "TCP Network Connection in"=w1265) -> ("TCP Command"=w1266:string, "TCP Network Connection out"=w1264:refnum<k5>, "Custom CMD?"=w1262:bool)  [unwired: 6 in, 1 out]
                  n550 = case shown="False" w1262 {
                    tunnel: w1266 -> [w1269 _]
                    tunnel: ["" ("Custom CMD State") "Post Setup Data" ("Custom CMD State")] -> w1261
                    frame False {
                      n551 = Spreadsheet String To Array(delimiter (Tab)=",", format string="%s", spreadsheet string=w1269, array type (2D Dbl)=string[][] []) -> (array=→"Chamber 3 Socket":string[][])
                    }
                    frame True {
                    }
                  }
                  n552 = local write "Custom CMD State"(w1261) -> ()
                }
                frame 3 {
                  n553 = call "RTS Read TCP Command.vi"("Client Side?"=TRUE, "TCP Network Connection in"=w1278) -> ("TCP Command"=w1279:string, "TCP Network Connection out"=w1277:refnum<k5>, "Custom CMD?"=w1275:bool)  [unwired: 6 in, 1 out]
                  n554 = case shown="False" w1275 {
                    tunnel: w1279 -> [w1282 _]
                    tunnel: ["" ("Custom CMD State") "Post Setup Data" ("Custom CMD State")] -> w1274
                    frame False {
                      n555 = Spreadsheet String To Array(delimiter (Tab)=",", format string="%s", spreadsheet string=w1282, array type (2D Dbl)=string[][] []) -> (array=→"Chamber 4 Socket":string[][])
                    }
                    frame True {
                    }
                  }
                  n556 = local write "Custom CMD State"(w1274) -> ()
                }
              }
            }
            frame True {
            }
          }
        }
        n557 = Bundle By Name(cluster=w1224, "Data.Clients"=w1221) -> (w1223:T65)
        n558 = call <vilib>:"Add State(s) to Queue__jki_lib_state_machine.vi"("State(s) in Front (\"\")"="Custom CMD State", "State(s) in (\"\")"=w1226) -> ("States Out"=w1225:string)  [unwired: 13 in]
      }
      frame "Update Values" {
        # "This is the listbox names\nwith the actual names..\nnot the custom"
        # "This is the custom data names (display only)"
        # "Allows automatic pause to plot\n(Easier for user to use)"
        n559 = Unbundle By Name(w1303) -> ("Tree Selection"=w1301:T1, "All Data"=w1302:dbl[][])
        n560 = local read "Chamber 1 Socket"() -> (w1300:string[][])
        n561 = local read "Chamber 2 Socket"() -> (w1299:string[][])
        n562 = local read "Chamber 3 Socket"() -> (w1298:string[][])
        n563 = local read "Chamber 4 Socket"() -> (w1297:string[][])
        n564 = call "RTS Update Values Both Save and No Save.vi"("All Data"=w1302, "error in"=w1306, "Chamber 1 Socket"=w1300, "Tree Selection"=w1301, "Chamber 2 Socket"=w1299, "Chamber 3 Socket"=w1298, "Chamber 4 Socket"=w1297) -> ("Point File Name"=w1288:string, "Chamber Data"=w1296:string[][], "Plot Data Array"=w1305:dbl[][], "Full Item Names"=w1295:string[], "Listbox Data"=w1292:string[][], "Custom Titles"=w1289:string[], "error out"=w1304:errorcluster)  [unwired: 6 in]
        n565 = case shown="True" "Update Plot" {
          tunnel: ["" ("State(s) in Front (\"\")") "Plot" ("State(s) in Front (\"\")")] -> w1308
          frame False {
          }
          frame True {
          }
        }
        n566 = Index Array(array=w1292, index (col)=0 ("disabled index (col)")) -> (element=w1290:string[])  [unwired: 1 in]
        n567 = Replace Array Subset(array=w1292, new element=w1289, index (col)=0 ("disabled index (col)")) -> (w1293:string[][])  [unwired: 1 in]
        n568 = property on="Configure Point File" class="Bool"("BoolText.Text"=w1288) -> ()  [unwired: 2 in, 2 out]
        n569 = Bundle By Name(cluster=w1303, "Chamber Data"=w1296, "All Data"=w1305, "Full Item Names"=w1295, "Listbox Item Names"=w1290, "Custom Titles"=w1289) -> (w1309:T65)
        n570 = property on="Listbox Data" class="MCListbox (strict)"("ItemNames"=w1293) -> ()  [unwired: 2 in, 2 out]
        n571 = call <vilib>:"Add State(s) to Queue__jki_lib_state_machine.vi"("State(s) in Front (\"\")"=w1308, "State(s) in (\"\")"=w1311) -> ("States Out"=w1310:string)  [unwired: 13 in]
      }
      frame "Contactor Settings" {
        n572 = Unbundle By Name(w1317) -> ("Chamber Data"=w1314:string[][])
        "Chamber Data" <- w1314
        n573 = call "RTS Extract Contactor Settings.vi"("Error In"=w1316, "Chamber 1 Socket"=w1314) -> ("Error Out"=w1315:errorcluster, "Current Contactor Settings"=→"Current Contactor Settings":T24, "Current Door Output Relays Status"=→"Current Door Output Relays Status":T25)  [unwired: 7 in]
        n574 = call <vilib>:"Add State(s) to Queue__jki_lib_state_machine.vi"("State(s) in (\"\")"=w1321) -> ("States Out"=w1320:string)  [unwired: 14 in]
      }
      frame "Write Server Data" {
        # "Send to the correct Server App"
        # "Reset the Write CMD\nfor the next CMD"
        n575 = Unbundle By Name(w1326) -> ("Data.Clients"=w1324:refnum<k5>[], "Server Write Data"=w1323:string)
        n576 = call "RTS Find TCP Socket to Send Too.vi"("Server Write Data"=w1323, "Clients"=w1324) -> ("TCP Send Socket"=w1322:refnum<k5>)  [unwired: 8 in, 1 out]
        n577 = Equal?(x=refnum<k5> refnum, y=w1322) -> (x = y?=w1329:bool)
        n578 = case shown="False" w1329 {
          tunnel: w1322 -> [w1343 _]
          tunnel: w1331 -> [w1339 w1344]
          tunnel: [w1342 w1344] -> w1328
          tunnel: w1323 -> [w1341 _]
          frame False {
            n579 = call "UTILITY Append Byte To Read TCP.vi"("Error In"=w1339, "Input String"=w1341) -> ("Error Out"=w1338:errorcluster, "Output String"=w1340:string)  [unwired: 8 in]
            n580 = TCP Write(connection ID=w1343, data in=w1340, error in (no error)=w1338) -> (error out=w1342:errorcluster)  [unwired: 3 out]
          }
          frame True {
          }
        }
        n581 = flat-sequence {
          tunnel: w1328 -> [w1337]
          tunnel: [w1337] -> w1327
          tunnel: w1326 -> [w1336]
          tunnel: [w1335] -> w1325
          frame #0 {
            n582 = Bundle By Name(cluster=w1336, "Server Write Data"="") -> (w1335:T65)
          }
        }
        n583 = call <vilib>:"Add State(s) to Queue__jki_lib_state_machine.vi"("State(s) in (\"\")"=w1333) -> ("States Out"=w1332:string)  [unwired: 14 in]
      }
      frame "Check Exit" {
        # "Need to populate the Save Status on the \"Station Settings\""
        # "Reads and processes server save state"
        n584 = Unbundle By Name(w1353) -> ("Tree Selection"=w1354:T1, "RTS Config Setup.Station Settings"=w1351:T12, "Station Owner Names"=w1357:string[], "CSV Data Save"=w1350:T31)
        n585 = local read "Chamber 1 Socket"() -> (w1364:string[][])
        n586 = local read "Chamber 2 Socket"() -> (w1363:string[][])
        n587 = local read "Chamber 3 Socket"() -> (w1362:string[][])
        n588 = local read "Chamber 4 Socket"() -> (w1361:string[][])
        n589 = local read "System Exit"() -> (w1365:bool)
        n590 = case shown="True" w1365 {
          tunnel: ["" "Macro: Exit"] -> w1366
          frame False {
          }
          frame True {
          }
        }
        n591 = call "RTS Start Stop Saving.vi"("Chamber 1 Socket"=w1364, "Chamber 2 Socket"=w1363, "CSV Data Save Input"=w1350, "Station Settings Input"=w1351, "Tree Selection"=w1354, "Chamber 3 Socket"=w1362, "Chamber 4 Socket"=w1361) -> ("Station Settings Output"=w1352:T12, "CSV Data Save Output"=w1349:T31, "Display"=w1360:string, "Current Status Display"=w1358:string[])  [unwired: 5 in, 4 out]
        n592 = Concatenate Strings(w1354, w1360) -> (w1346:string)
        "Tree Selection Display" <- w1346
        n593 = Build Array(w1358, w1357) -> (w1356:string[][])
        n594 = Transpose 2D Array(2D array=w1356) -> (transposed array=w1355:string[][])
        n595 = property on="Save Data" class="Bool (strict)"("BoolText.Text"=w1346) -> ()  [unwired: 2 in, 2 out]
        n596 = property on="Room Status" class="MCListbox (strict)"("ItemNames"=w1355, "ColHdrString"=string[] ["Room Status", "Owner"] ("Row Header Strings[]")) -> ()  [unwired: 2 in, 2 out]
        n597 = Bundle By Name(cluster=w1353, "RTS Config Setup.Station Settings"=w1352, "CSV Data Save"=w1349) -> (w1348:T65)
        n598 = Unbundle By Name(w1348) -> ("RTS Config Setup"=w1347:T6, "RTS Config Setup.Station Settings.Save Status"=→"Save Status":T13)
        n599 = call <vilib>:"Add State(s) to Queue__jki_lib_state_machine.vi"("State(s) in Front (\"\")"=w1366, "State(s) in (\"\")"=w1369) -> ("States Out"=w1368:string)  [unwired: 13 in]
        n600 = local write "RTS Config Setup Output"(w1347) -> ()
        n601 = local write "CSV Data Save"(w1349) -> ()
      }
      frame "Tree Selection Read" {
        n602 = Unbundle By Name(w1373) -> ("CSV Data Save"=w1377:T31, "Tree Selection"=w1372:T1)
        n603 = case shown="\"1-1\", \"2-1\", \"3-1\", \"4-1\"" w1372 {
          tunnel: w1373 -> [_ w1410 w1412 w1414 w1416 w1418 w1420 w1422 w1424]
          tunnel: [FALSE ("Save Status 8") w1409 w1411 w1413 w1415 w1417 w1419 w1421 w1423] -> w1385
          frame Default {
          }
          frame "1-1", "2-1", "3-1", "4-1" {
            n604 = Unbundle By Name(w1410) -> ("RTS Config Setup.Station Settings.Save Status.Save Status 1"=w1409:bool)
          }
          frame "1-2", "2-2", "3-2", "4-2" {
            n605 = Unbundle By Name(w1412) -> ("RTS Config Setup.Station Settings.Save Status.Save Status 2"=w1411:bool)
          }
          frame "1-3", "2-3", "3-3", "4-3" {
            n606 = Unbundle By Name(w1414) -> ("RTS Config Setup.Station Settings.Save Status.Save Status 3"=w1413:bool)
          }
          frame "1-4", "2-4", "3-4", "4-4" {
            n607 = Unbundle By Name(w1416) -> ("RTS Config Setup.Station Settings.Save Status.Save Status 4"=w1415:bool)
          }
          frame "1-5", "2-5", "3-5", "4-5" {
            n608 = Unbundle By Name(w1418) -> ("RTS Config Setup.Station Settings.Save Status.Save Status 5"=w1417:bool)
          }
          frame "1-6", "2-6", "3-6", "4-6" {
            n609 = Unbundle By Name(w1420) -> ("RTS Config Setup.Station Settings.Save Status.Save Status 6"=w1419:bool)
          }
          frame "1-7", "2-7", "3-7", "4-7" {
            n610 = Unbundle By Name(w1422) -> ("RTS Config Setup.Station Settings.Save Status.Save Status 7"=w1421:bool)
          }
          frame "1-8", "2-8", "3-8", "4-8" {
            n611 = Unbundle By Name(w1424) -> ("RTS Config Setup.Station Settings.Save Status.Save Status 8"=w1423:bool)
          }
        }
        n612 = local read "Chamber 1 Socket"() -> (w1383:string[][])
        n613 = local read "Chamber 2 Socket"() -> (w1382:string[][])
        n614 = local read "Chamber 3 Socket"() -> (w1381:string[][])
        n615 = local read "Chamber 4 Socket"() -> (w1380:string[][])
        n616 = case shown="True" w1385 {
          tunnel: w1375 -> [w1398 w1407]
          tunnel: [w1397 w1406] -> w1379
          tunnel: [w1390 w1405] -> w1384
          tunnel: w1372 -> [w1396 w1404]
          tunnel: w1377 -> [_ w1403]
          tunnel: w1383 -> [w1395 w1402]
          tunnel: w1382 -> [w1394 w1401]
          tunnel: w1381 -> [w1393 w1400]
          tunnel: w1380 -> [w1392 w1399]
          frame False {
            n617 = call "RTS TCP Real Time.vi"("Chamber 1 Socket"=w1395, "All Data in"=dbl[][] [] ("Station Data"), "Chamber 2 Socket"=w1394, "Chamber 3 Socket"=w1393, "error in (no error)"=w1398, "Chamber 4 Socket"=w1392, "Tree Selection"=w1396) -> ("All Data out"=w1390:dbl[][], "error out"=w1397:errorcluster)  [unwired: 2 in, 5 out]
          }
          frame True {
            n618 = call "RTS Get TDMS Data.vi"("CSV Data Save"=w1403, "Chamber 1 Socket"=w1402, "Chamber 2 Socket"=w1401, "Chamber 3 Socket"=w1400, "Chamber 4 Socket"=w1399, "error in (no error)"=w1407, "Tree Selection"=w1404) -> ("Station Data"=w1405:dbl[][], "error out"=w1406:errorcluster)  [unwired: 10 in, 1 out]
          }
        }
        n619 = flat-sequence {
          tunnel: w1379 -> [w1389]
          tunnel: [w1389] -> w1374
          tunnel: [w1388] -> w1378
          frame #0 {
            w1388 = i32[] [] ("ListBox Selection")
            n620 = property on="Multicolumn Listbox" class="MCListbox (strict)"("Value"=w1388) -> ()  [unwired: 2 in, 2 out]
          }
        }
        n621 = call <vilib>:"Add State(s) to Queue__jki_lib_state_machine.vi"("State(s) in (\"\")"=w1386) -> ("States Out"=w1387:string)  [unwired: 14 in]
        n622 = Bundle By Name(cluster=w1373, "All Data"=w1384, "ListBox Selection"=w1378) -> (w1376:T65)
      }
    }
    n623 = case shown="True" "Debug?" {
      tunnel: w759 -> [w770 w773]
      tunnel: w758 -> [_ w772]
      tunnel: [w770 w771] -> w757
      frame False {
      }
      frame True {
        n624 = Build Array (concatenate)(w773, w772) -> (w771:string[])
        "Debug array" <- w771
      }
    }
  }
  "Error Out" <- w17
  n625 = call "RTS Parse Setup File.vi"() -> ()  [unwired: 9 in, 3 out]
  n626 = call "RTS Parse Setup File.vi"() -> ()  [unwired: 9 in, 3 out]
